vi "OP_Print_TPS_cluster_20170807.vi"() -> ()   [LabVIEW 2013]
uses:
  <userlib>/caLab/Private/Get_PV-1D.vi
  <userlib>/caLab/Private/Get_PV.vi
panel:
  out "x = y?":bool
  out "NOW time":string
  out "NOW date":string
  out "loop2":i32=243
  in  "Save Button":bool
  out "error out 3":errorcluster
  in  "stop":bool
  out "time kickeron":string="kickers"
  out "date kickeron":string="wait to fire"
  out "Cluster":T1={"SR Fill Pattern"=array[864 elements], "Beam Current(mA"=301.91562200000004, "Beam Lifetime(min)"=669.1065769463743, "Beamsize X(um)"=55.54579477590784, "Beamsize Y(um)"=33.648665625479325, "Tune X(from BPM)"=0.1399, "Tune Y(from BPM)"=0.14, "Mode"="Top-Up", "NuX(from BBF) "=0.16718639681347974, "NuY(from BBF)"=0.25219386232318686, "IU22-23gap(R)"=11.0, "IU22-05gap(R)"=7.558, "IU22-05M"=TRUE, "IU22A-09gap(R)"=8.075, "IU22A-09M"=TRUE, "IU22B-09gap(R)"=40.001, "IU22B-09M"=FALSE, "IUT22-21gap(R)"=7.0, "IUT22-21M"=TRUE, "IU22-23M"=TRUE, "IU22A-25gap(R)"=8.18, "IU22A-25M"=TRUE, "IU22B-25gap(R)"=40.0, "IU22B-25M"=FALSE, "EPU48A-41gap(R)"=64.99985000000001, "EPU48A-41gM"=TRUE, "EPU48B-41gap(R)"=65.00399999999999, "EPU48B-41gM"=FALSE, "EPU46-45gap(R)"=45.00005, "EPU46-45gM"=TRUE, "EPU48A-41phase(R)"=0.0001, "EPU48B-41phase(R)"=0.00055, "EPU46-45phase(R)"=0.0, "Grid volt.(V)(S)"=33.0, "Gun mode"="MBM", "Mod.3 HV(kV)(S)"=35.800000000000026, "SR"="SR_DMB_2016_1102_1124LOCO.data", "BR"="Booster_JT_2016_1005_1200.data", "Linac"="Linac2016_1005_0935.data", "LTB"="LTB_JT_2016_1005_1200.data", "BTS"="BTS_2016_1116_1020.data", "RF2 remote"=TRUE, "RF2 OP mode"=TRUE, "RF2 phase.(S)"=-56.70000000000001, "RF Freq.(s)"=499654660.62238467, "RF2 gap volt.(S)"=1400.0, "RF3 remote"=TRUE, "RF3 OP mode"=TRUE, "RF3 phase.(S)"=160.0, "RF3 gap volt.(S)"=1400.0, "BBF V"=TRUE, "BBF H"=TRUE, "BR ext. kicker1(kV)"=18.266, "BR ext. kicker2(kV)"=18.26600000000001, "BR ext. sep.1(V)"=318.8444, "BR ext. sep.2(V)"=444.5, "BR inj. sep.(V)"=105.2, "BR inj. kicker(kV)"=16.40000000000001, "SR kicker4(kV)"=8.27, "SR kicker3(kV)"=8.315, "SR kicker2(kV)"=8.325, "SR kicker1(kV)"=8.4, "SR inj. sep.2(V)"=417.0, "SR inj. sep.1(V)"=419.3416, "Bucket Start"=100.0, "Bucket Last"=630.0, "Bucket Step"=10.0, "Orbit ILK(P)"=TRUE, "IU22-05 Hutch Enable"=TRUE, "IU22A-09M Hutch Enable"=TRUE, "IUT22-21M Hutch Enable"=TRUE, "IU22-23M Hutch Enable"=FALSE, "IU22A-25M Hutch Enable"=TRUE, "EPU48A-41M Hutch Enable"=FALSE, "EPU46-45M Hutch Enable"=TRUE, "EPU46-45 FE Enable"=TRUE, "EPU48A-41 FE Enable"=FALSE, "IU22A-25 FE Enable"=TRUE, "IU22-23 FE Enable"=FALSE, "IUT22-21 FE Enable"=TRUE, "IU22A-09 FE Enable"=TRUE, "IU22-05 FE Enable"=TRUE, "EPU48A-41pM"=TRUE, "EPU48B-41pM"=FALSE, "EPU46-45pM"=FALSE, "Gun volt.(V)(S)"=23.5, "Width count"=30.0, "2ns step"=0.0, "10ps delay"=100.0, "phase shifter"=130.00060000000002, "Taper"=-1.0899999999999999, "05XBPMX 1"=115.877, "09XBPMX 1"=471.421, "21XBPMX 1"=612.331, "23XBPMX 1"=-46.736000000000004, "25XBPMX 1"=462.29900000000004, "41XBPMX 1"=364.139, "45XBPMX 1"=-164.196, "05XBPMY 1"=-62.875, "09XBPMY 1"=-23.034, "21XBPMY 1"=-27.449, "23XBPMY 1"=-89.72200000000001, "25XBPMY 1"=459.291, "41XBPMY 1"=-111.624, "45XBPMY 1"=-57.689, "FOFB H"="On", "FOFB V"="On", "time string"="21:36:25", "date"="2016/11/21", "date (last kicker ON)"="wait to fire", "time string (last kicker ON)"="", "BPMX Graph"={[1, 2, 3, 4, 5, 6, 7, 8, 9, 10, 11, 12, 13, 14, 15, 16, 17, 18, 19, 20, 21, 22, 23, 24, 25, 26, 27, 28, 29, 30, 31, 32, 33, 34, 35, 36, 37, 38, 39, 40, 41, 42, 43, 44, 45, 46, 47, 48, 49, 50, 51, 52, 53, 54, 55, 56, 57, 58, 59, 60, 61, 62, 63, 64, 65, 66, 67, 68, 69, 70, 71, 72, 73, 74, 75, 76, 77, 78, 79, 80, 81, 82, 83, 84, 85, 86, 87, 88, 89, 90, 91, 92, 93, 94, 95, 96, 97, 98, 99, 100, 101, 102, 103, 104, 105, 106, 107, 108, 109, 110, 111, 112, 113, 114, 115, 116, 117, 118, 119, 120, 121, 122, 123, 124, 125, 126, 127, 128, 129, 130, 131, 132, 133, 134, 135, 136, 137, 138, 139, 140, 141, 142, 143, 144, 145, 146, 147, 148, 149, 150, 151, 152, 153, 154, 155, 156, 157, 158, 159, 160, 161, 162, 163, 164, 165, 166, 167, 168, 169, 170, 171, 172, 173, 174], "1rst Value (number)"=[-31.198, -3.303, -73.172, -2.032, 86.386, -75.851, 71.519, -46.03, 6.824, -37.804, 68.275, -4.672, -223.404, -16.867, -6.964, -259.448, -62.697, 1.8880000000000001, 75.267, -92.668, 86.714, -30.843, 12.767, -107.398, -44.436, 161.126, 208.922, 211.488, -27.247, 79.489, 826.962, 470.705, -115.522, -41.497, 159.486, -54.261, -0.64, 42.641, -2.466, -143.394, -24.785, 138.912, -65.805, 42.325, 32.891, -7.298, -96.724, -31.725, 98.531, -80.64, 64.163, 94.83, -44.03, -163.192, 50.589, 46.669000000000004, -87.508, 78.479, 31.618000000000002, -17.077, -125.32600000000001, -3.845, 98.34100000000001, -39.679, 50.247, -58.208, 40.297000000000004, -69.857, 42.548, -19.403, -211.0, -9.082, -322.597, -233.847, -140.75, 97.087, -15.869, -29.053, 59.46, -115.316, 70.896, -60.685, 33.715, 12.09, -520.422, -138.423, -302.753, 79.862, 120.014, 122.671, -55.812, 27.084, 39.115, -138.936, 156.631, 53.777, -72.647, -52.588, 16.002, 45.197, -117.489, 121.709, 27.952, -31.609, -113.58500000000001, 45.019, 55.136, -130.553, 138.93200000000002, 35.998, -30.631, -96.529, -7.589, 100.395, -93.919, 40.569, 79.538, -68.044, -134.578, 2.52, 84.539, -59.166000000000004, 42.576, 34.657000000000004, -15.805, -52.158, 18.484, 4.346, -157.404, 182.672, 202.518, -164.868, -53.871, 8.066, -9.738, -55.594, 92.623, -13.785, 11.587, -60.627, -47.704, 65.516, 57.924, 148.347, -201.348, -302.753, 189.117, 72.681, -134.928, 39.791000000000004, 45.938, -49.072, 54.473, 28.991, -20.657, -80.283, -20.264, 106.907, -121.271, 150.281, -2.243, -11.844, -122.82300000000001, 0.973, 114.186, -107.94, 95.485, 40.314, -36.956, -134.537, 16.196, 91.88, -35.505, -0.018000000000000002]}, "BPMY Graph"={[1, 2, 3, 4, 5, 6, 7, 8, 9, 10, 11, 12, 13, 14, 15, 16, 17, 18, 19, 20, 21, 22, 23, 24, 25, 26, 27, 28, 29, 30, 31, 32, 33, 34, 35, 36, 37, 38, 39, 40, 41, 42, 43, 44, 45, 46, 47, 48, 49, 50, 51, 52, 53, 54, 55, 56, 57, 58, 59, 60, 61, 62, 63, 64, 65, 66, 67, 68, 69, 70, 71, 72, 73, 74, 75, 76, 77, 78, 79, 80, 81, 82, 83, 84, 85, 86, 87, 88, 89, 90, 91, 92, 93, 94, 95, 96, 97, 98, 99, 100, 101, 102, 103, 104, 105, 106, 107, 108, 109, 110, 111, 112, 113, 114, 115, 116, 117, 118, 119, 120, 121, 122, 123, 124, 125, 126, 127, 128, 129, 130, 131, 132, 133, 134, 135, 136, 137, 138, 139, 140, 141, 142, 143, 144, 145, 146, 147, 148, 149, 150, 151, 152, 153, 154, 155, 156, 157, 158, 159, 160, 161, 162, 163, 164, 165, 166, 167, 168, 169, 170, 171, 172, 173, 174], "1rst Value (number)"=[-99.743, 2.851, -30.024, 83.777, -46.733000000000004, -39.889, 2.349, -4.944, 17.022000000000002, 9.824, 11.632, 41.188, -13.992, 13.911, -6.211, 53.857, -48.993, -32.789, -6.3740000000000006, -62.867000000000004, -8.332, 72.09400000000001, -75.398, 53.283, 63.008, -2.23, 43.024, 32.073, -246.641, -93.162, 456.41700000000003, 88.299, 58.803000000000004, 1.7590000000000001, 35.664, 6.575, 18.59, -30.439, 11.254, -28.256, -62.707, -4.503, 1.31, -21.571, 34.77, -8.876, 31.237000000000002, 25.402, 2.726, 20.655, -7.845, -1.443, -31.935000000000002, -16.981, 13.022, 17.515, -82.867, 61.285000000000004, -57.573, 110.363, -27.753, 28.322, -9.241, 53.929, -25.816, 24.231, -57.876, -11.578, 32.087, -70.84, 64.43, 9.409, -157.639, -57.0, 39.267, 30.23, 18.993000000000002, -33.97, 26.195, -10.585, -17.617, -18.667, 31.615000000000002, -25.437, 29.564, 13.537, 6.728, 163.38400000000001, 106.51, -70.056, 12.874, -4.125, -10.855, -21.856, 1.947, 8.096, 11.402000000000001, 5.761, 41.929, -8.752, 18.634, 7.553, -40.034, 39.183, -25.067, -32.557, 5.393, -17.564, -1.614, 20.498, -14.818, 10.313, 35.254, -35.886, 58.359, -36.56, -20.354, 7.593, -21.256, -8.001, -16.79, 10.18, -16.327, 20.416, -10.539, 19.944, -6.801, 13.068, -13.644, 3.468, -0.983, -17.6, 6.785, -26.101, -11.52, 61.191, -32.777, 13.536, 4.026, -14.682, 52.057, -53.883, 27.118000000000002, 31.672, 79.62, 17.715, 15.693, 113.157, -57.095, 14.214, -4.787, -11.148, -3.157, -6.251, -0.764, 3.563, 7.3500000000000005, 10.779, 21.129, 11.36, 7.771, -14.787, -13.278, 0.279, -13.516, -62.422000000000004, -13.389000000000001, 80.56400000000001, -108.465, 69.885, 30.116, 21.421, 32.779, -10.527000000000001]}, "Radio Buttons 2"=enum."absolute", "09XBPMX 2"="", "09XBPMY 2"="", "05XBPMY 2"="", "05XBPMX 2"="", "21XBPMY 2"="", "21XBPMX 2"="", "23XBPMY 2"="", "23XBPMX 2"="", "25XBPMY 2"="", "25XBPMX 2"="", "41XBPMY 2"="", "41XBPMX 2"="", "45XBPMX 2"="", "45XBPMY 2"="", "05 mode"="", "09A mode"="", "09B mode"="", "21 mode"="", "23 mode"="", "25A mode"="", "25B mode"="", "41A mode"="", "41B mode"="", "46 mode"=""} {"45XBPMY 1" format="%#.2f"; "41XBPMY 1" format="%#.2f"; "25XBPMY 1" format="%#.2f"; "23XBPMY 1" format="%#.2f"; "21XBPMY 1" format="%#.2f"; "09XBPMY 1" format="%#.2f"; "05XBPMY 1" format="%#.2f"; "45XBPMX 1" format="%#.2f"; "41XBPMX 1" format="%#.2f"; "25XBPMX 1" format="%#.2f"; "23XBPMX 1" format="%#.2f"; "21XBPMX 1" format="%#.2f"; "09XBPMX 1" format="%#.2f"; "05XBPMX 1" format="%#.2f"; "Taper" format="%#.4f"; "phase shifter" format="%#.3f"; "10ps delay" format="%#.1f"; "2ns step" format="%#.1f"; "Width count" format="%#.1f"; "Gun volt.(V)(S)" format="%#.1f"; "Bucket Step" format="%#.2f"; "Bucket Last" format="%#.2f"; "Bucket Start" format="%#.2f"; "BR ext. kicker1(kV)" format="%#.2f"; "BR ext. kicker2(kV)" format="%#.2f"; "BR ext. sep.1(V)" format="%#.2f"; "BR ext. sep.2(V)" format="%#.2f"; "BR inj. sep.(V)" format="%#.3f"; "BR inj. kicker(kV)" format="%#.3f"; "SR kicker4(kV)" format="%#.2f"; "SR kicker3(kV)" format="%#.2f"; "SR kicker2(kV)" format="%#.2f"; "SR kicker1(kV)" format="%#.2f"; "SR inj. sep.2(V)" format="%#.2f"; "SR inj. sep.1(V)" format="%#.2f"; "RF3 gap volt.(S)" format="%#.0f"; "RF3 phase.(S)" format="%#.1f"; "RF2 gap volt.(S)" format="%#.0f"; "RF Freq.(s)" format="%#.1f"; "RF2 phase.(S)" format="%#.1f"; "Mod.3 HV(kV)(S)" format="%#.3f"; "Grid volt.(V)(S)" format="%#.1f"; "EPU46-45phase(R)" format="%#.4f"; "EPU48B-41phase(R)" format="%#.4f"; "EPU48A-41phase(R)" format="%#.4f"; "EPU46-45gap(R)" format="%#.4f"; "EPU48B-41gap(R)" format="%#.4f"; "EPU48A-41gap(R)" format="%#.4f"; "IU22B-25gap(R)" format="%#.4f"; "IU22A-25gap(R)" format="%#.4f"; "IUT22-21gap(R)" format="%#.4f"; "IU22B-09gap(R)" format="%#.4f"; "IU22A-09gap(R)" format="%#.4f"; "IU22-05gap(R)" format="%#.4f"; "IU22-23gap(R)" format="%#.4f"; "NuY(from BBF)" format="%#.4f"; "NuX(from BBF)" format="%#.4f"; "Tune Y(from BPM)" format="%#.4f"; "Tune X(from BPM)" format="%#.4f"; "Beamsize Y(um)" format="%#.2f"; "Beamsize X(um)" format="%#.2f"; "Beam Lifetime(min)" format="%#.3f"; "Beam Current(mA" format="%#.3f"}
  out "date (last Gun ON)":string="2016/08/29"
  out "time string (last Gun ON)":string="23:28:50"
  out "Value Array (number) 7":dbl[](array[numeric])=[115.877, -62.875, 471.421, -23.034, 612.331, -27.449, -46.736000000000004, -89.72200000000001, 462.29900000000004, 459.291, 364.139, -111.624, -164.196, -57.689]
  out "Value Array (number) 6":dbl[](array[numeric])=[7.558, 8.075, 40.001, 7.0, 11.0, 8.18, 40.0, 64.99985000000001, 0.0001, 65.00399999999999, 0.00055, 45.00005, 0.0, -1.0899999999999999, 130.00060000000002]
  out "1rst Value (string) 2":string[](array[string])=["MBM", "33", "23.5", "350", "35.8", "22485", "22485", "62", "30", "0", "0", "160", "100"]
  out "Value Array (number) 5":dbl[](array[numeric])=[499654641.19275105, 1.0, 0.0, 1335.005102558433, 1400.0, -56.1, 1.0, 0.0, 1362.1066276040413, 1400.0, 160.0]
  out "1rst Value (string)":string[](array[string])=["Linac2016_1005_0935.data", "LTB_JT_2016_1005_1200.data", "Booster_JT_2016_1005_1200.data", "BTS_2016_1116_1020.data", "SR_DMB_2016_1102_1124LOCO.data"]
  out "Value Array (number) 4":dbl[](array[numeric])=[499654660.62238467, 1.0, 0.0, 1334.266859115235, 1400.0, -56.70000000000001, 1.0, 0.0, 1364.570619451613, 1400.0, 160.0]
  out "Value Array (number) 3":dbl[](array[numeric])=[0.0, 33.0, 23.5, 350.0, 35.800000000000026, 22485.0, 22485.0, 62.0, 30.0, 0.0, 0.0, 160.0, 100.0]
  out "Value Array (number) 2":dbl[](array[numeric])=[105.2, 16.40000000000001, 18.266, 18.26600000000001, 318.8444, 444.5, 419.3416, 417.0, 8.4, 8.325, 8.315, 8.27]
  out "Value Array (number)":dbl[](array[numeric])=[1.0, 301.91562200000004, 669.1065769463743, 46.211143740355936, 27.993898190914578, 0.11937377690802348, 0.2162426614481409, 96.68439483642578, 145.84446716308594, 100.0, 630.0, 10.0]
  out "Orbit ILK(A)":bool
  out "Orbit INT. Ang Active":bool
  out "Orbit INT.Ang. On":bool
  out "Orbit INT. Pos Active":bool
  out "Orbit INT.Pos. On":bool
  out "SBM volt.(S)":dbl=350.0 format="%#.1f"
  out "MBM volt.(S)":dbl=23.5 format="%#.1f"
  in  "Copy Button":bool
  in  "Print Button":bool
  in  "Help Button":bool
  in  "Refresh Button":bool
  in  "Open Button":bool
  out "Gun WCM":dbl[](graph)
  out "BR Fill Pattern":dbl[](graph)
  # "TPS OP Handover Information"
  # "Others"
  # "Time："
  # "Valve  Status"
  # "follow"
  # "SM Status"
  # "歷史電流圖\ntrip次數?\n輻射劑量?\n平均氣壓\n目前最高累計劑量\n最近一次觸發時BR電流及WCM數值"
  # "TPS Operational Handover Information v1.2"
  # "SR Status"
  # "Feedback"
  # "Pulse Mag"
  # "LINAC"
  # "x8(ns)"
  # "x2(ns)"
  # "x0.01(ns)"
  # "RF Status"
  # "Hz"
  # "(kV)"
  # "(kV)"
  # "Changeliang@LOP.NSRRC"
  # "SR Fill Pattern"
  # "Lattice Files in using"
  # "ID &Beamline (R)"
  # "mode"
  # "Gap\nmm"
  # "Motor"
  # "Phase"
  # "FE/Hutch"
  # "phase\nshifter"
  # "Taper\n(enc)"
  # "XBPM1X\num"
  # "XBPM1Y\num"
  # "XBPM2X\num"
  # "XBPM2Y\num"
  # "05"
  # "09"
  # "21"
  # "23"
  # "25"
  # "41"
  # "45"
  # "SR Orbit"
  # "BPMX"
  # "BPMY"
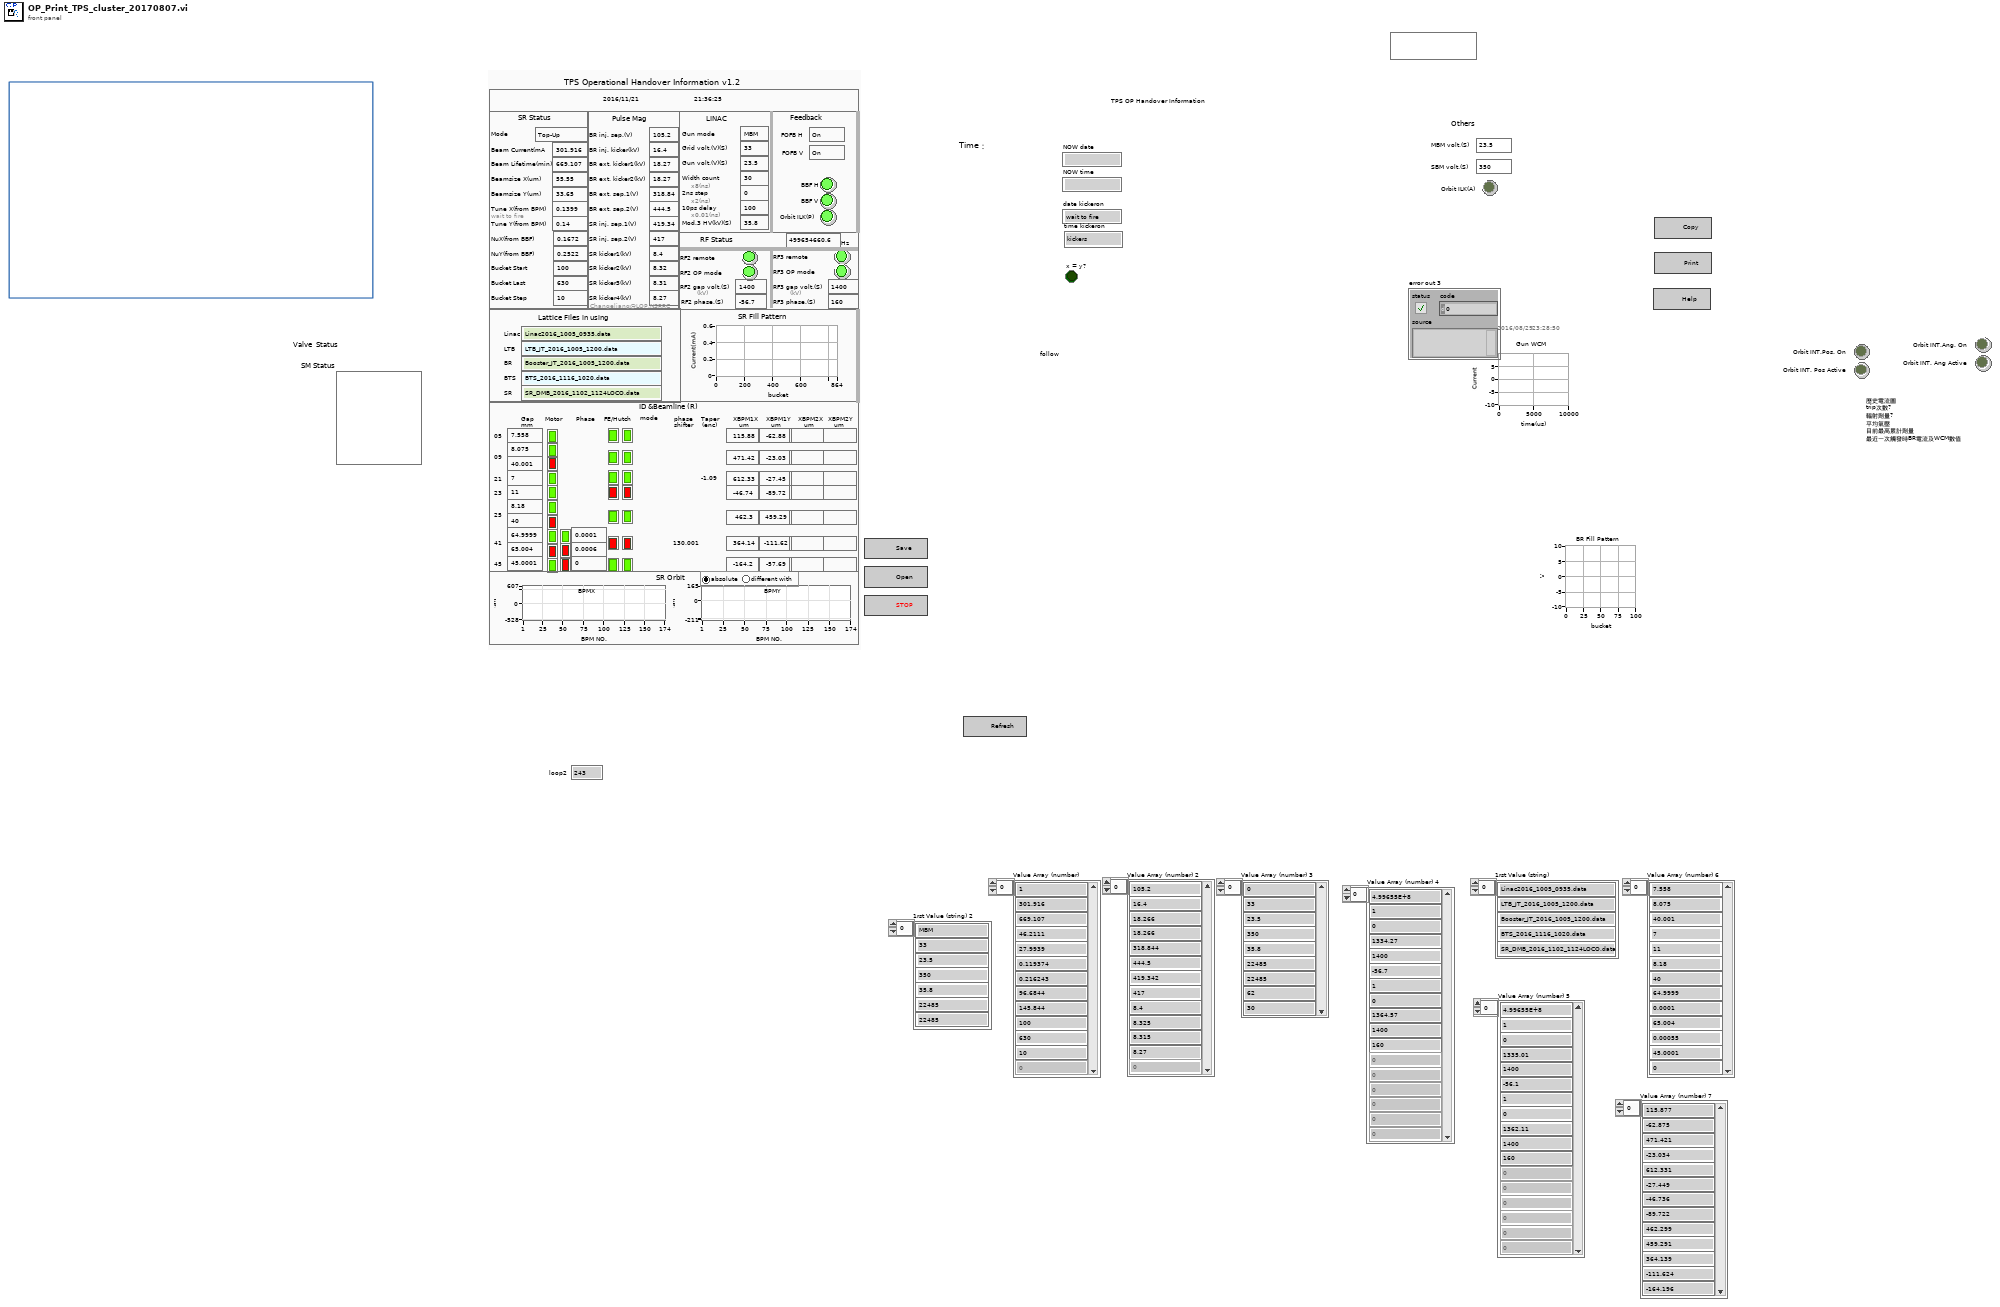
[diagram p1: front panel]
types:
  T1 = cluster{"SR Fill Pattern":dbl[], "Beam Current(mA":dbl, "Beam Lifetime(min)":dbl, "Beamsize X(um)":dbl, "Beamsize Y(um)":dbl, "Tune X(from BPM)":dbl, "Tune Y(from BPM)":dbl, "Mode":string, "NuX(from BBF) ":dbl, "NuY(from BBF)":dbl, "IU22-23gap(R)":dbl, "IU22-05gap(R)":dbl, "IU22-05M":bool, "IU22A-09gap(R)":dbl, "IU22A-09M":bool, "IU22B-09gap(R)":dbl, "IU22B-09M":bool, "IUT22-21gap(R)":dbl, "IUT22-21M":bool, "IU22-23M":bool, "IU22A-25gap(R)":dbl, "IU22A-25M":bool, "IU22B-25gap(R)":dbl, "IU22B-25M":bool, "EPU48A-41gap(R)":dbl, "EPU48A-41gM":bool, "EPU48B-41gap(R)":dbl, "EPU48B-41gM":bool, "EPU46-45gap(R)":dbl, "EPU46-45gM":bool, "EPU48A-41phase(R)":dbl, "EPU48B-41phase(R)":dbl, "EPU46-45phase(R)":dbl, "Grid volt.(V)(S)":dbl, "Gun mode":string, "Mod.3 HV(kV)(S)":dbl, "SR":string, "BR":string, "Linac":string, "LTB":string, "BTS":string, "RF2 remote":bool, "RF2 OP mode":bool, "RF2 phase.(S)":dbl, "RF Freq.(s)":dbl, "RF2 gap volt.(S)":dbl, "RF3 remote":bool, "RF3 OP mode":bool, "RF3 phase.(S)":dbl, "RF3 gap volt.(S)":dbl, "BBF V":bool, "BBF H":bool, "BR ext. kicker1(kV)":dbl, "BR ext. kicker2(kV)":dbl, "BR ext. sep.1(V)":dbl, "BR ext. sep.2(V)":dbl, "BR inj. sep.(V)":dbl, "BR inj. kicker(kV)":dbl, "SR kicker4(kV)":dbl, "SR kicker3(kV)":dbl, "SR kicker2(kV)":dbl, "SR kicker1(kV)":dbl, "SR inj. sep.2(V)":dbl, "SR inj. sep.1(V)":dbl, "Bucket Start":dbl, "Bucket Last":dbl, "Bucket Step":dbl, "Orbit ILK(P)":bool, "IU22-05 Hutch Enable":bool, "IU22A-09M Hutch Enable":bool, "IUT22-21M Hutch Enable":bool, "IU22-23M Hutch Enable":bool, "IU22A-25M Hutch Enable":bool, "EPU48A-41M Hutch Enable":bool, "EPU46-45M Hutch Enable":bool, "EPU46-45 FE Enable":bool, "EPU48A-41 FE Enable":bool, "IU22A-25 FE Enable":bool, "IU22-23 FE Enable":bool, "IUT22-21 FE Enable":bool, "IU22A-09 FE Enable":bool, "IU22-05 FE Enable":bool, "EPU48A-41pM":bool, "EPU48B-41pM":bool, "EPU46-45pM":bool, "Gun volt.(V)(S)":dbl, "Width count":dbl, "2ns step":dbl, "10ps delay":dbl, "phase shifter":dbl, "Taper":dbl, "05XBPMX 1":dbl, "09XBPMX 1":dbl, "21XBPMX 1":dbl, "23XBPMX 1":dbl, "25XBPMX 1":dbl, "41XBPMX 1":dbl, "45XBPMX 1":dbl, "05XBPMY 1":dbl, "09XBPMY 1":dbl, "21XBPMY 1":dbl, "23XBPMY 1":dbl, "25XBPMY 1":dbl, "41XBPMY 1":dbl, "45XBPMY 1":dbl, "FOFB H":string, "FOFB V":string, "time string":string, "date":string, "date (last kicker ON)":string, "time string (last kicker ON)":string, "BPMX Graph":cluster{i32[], "1rst Value (number)":dbl[]}, "BPMY Graph":cluster{i32[], "1rst Value (number)":dbl[]}, "Radio Buttons 2":enum32{"absolute", "different with"}, "09XBPMX 2":string, "09XBPMY 2":string, "05XBPMY 2":string, "05XBPMX 2":string, "21XBPMY 2":string, "21XBPMX 2":string, "23XBPMY 2":string, "23XBPMX 2":string, "25XBPMY 2":string, "25XBPMX 2":string, "41XBPMY 2":string, "41XBPMX 2":string, "45XBPMX 2":string, "45XBPMY 2":string, "05 mode":string, "09A mode":string, "09B mode":string, "21 mode":string, "23 mode":string, "25A mode":string, "25B mode":string, "41A mode":string, "41B mode":string, "46 mode":string}
  T2 = typedef "imagedata.ctl" = cluster{"image type":i32, "image depth":i32, "image":u8[], "mask":u8[], "colors":u32[], "Rectangle":cluster{"left":i16, "top":i16, "right":i16, "bottom":i16}}
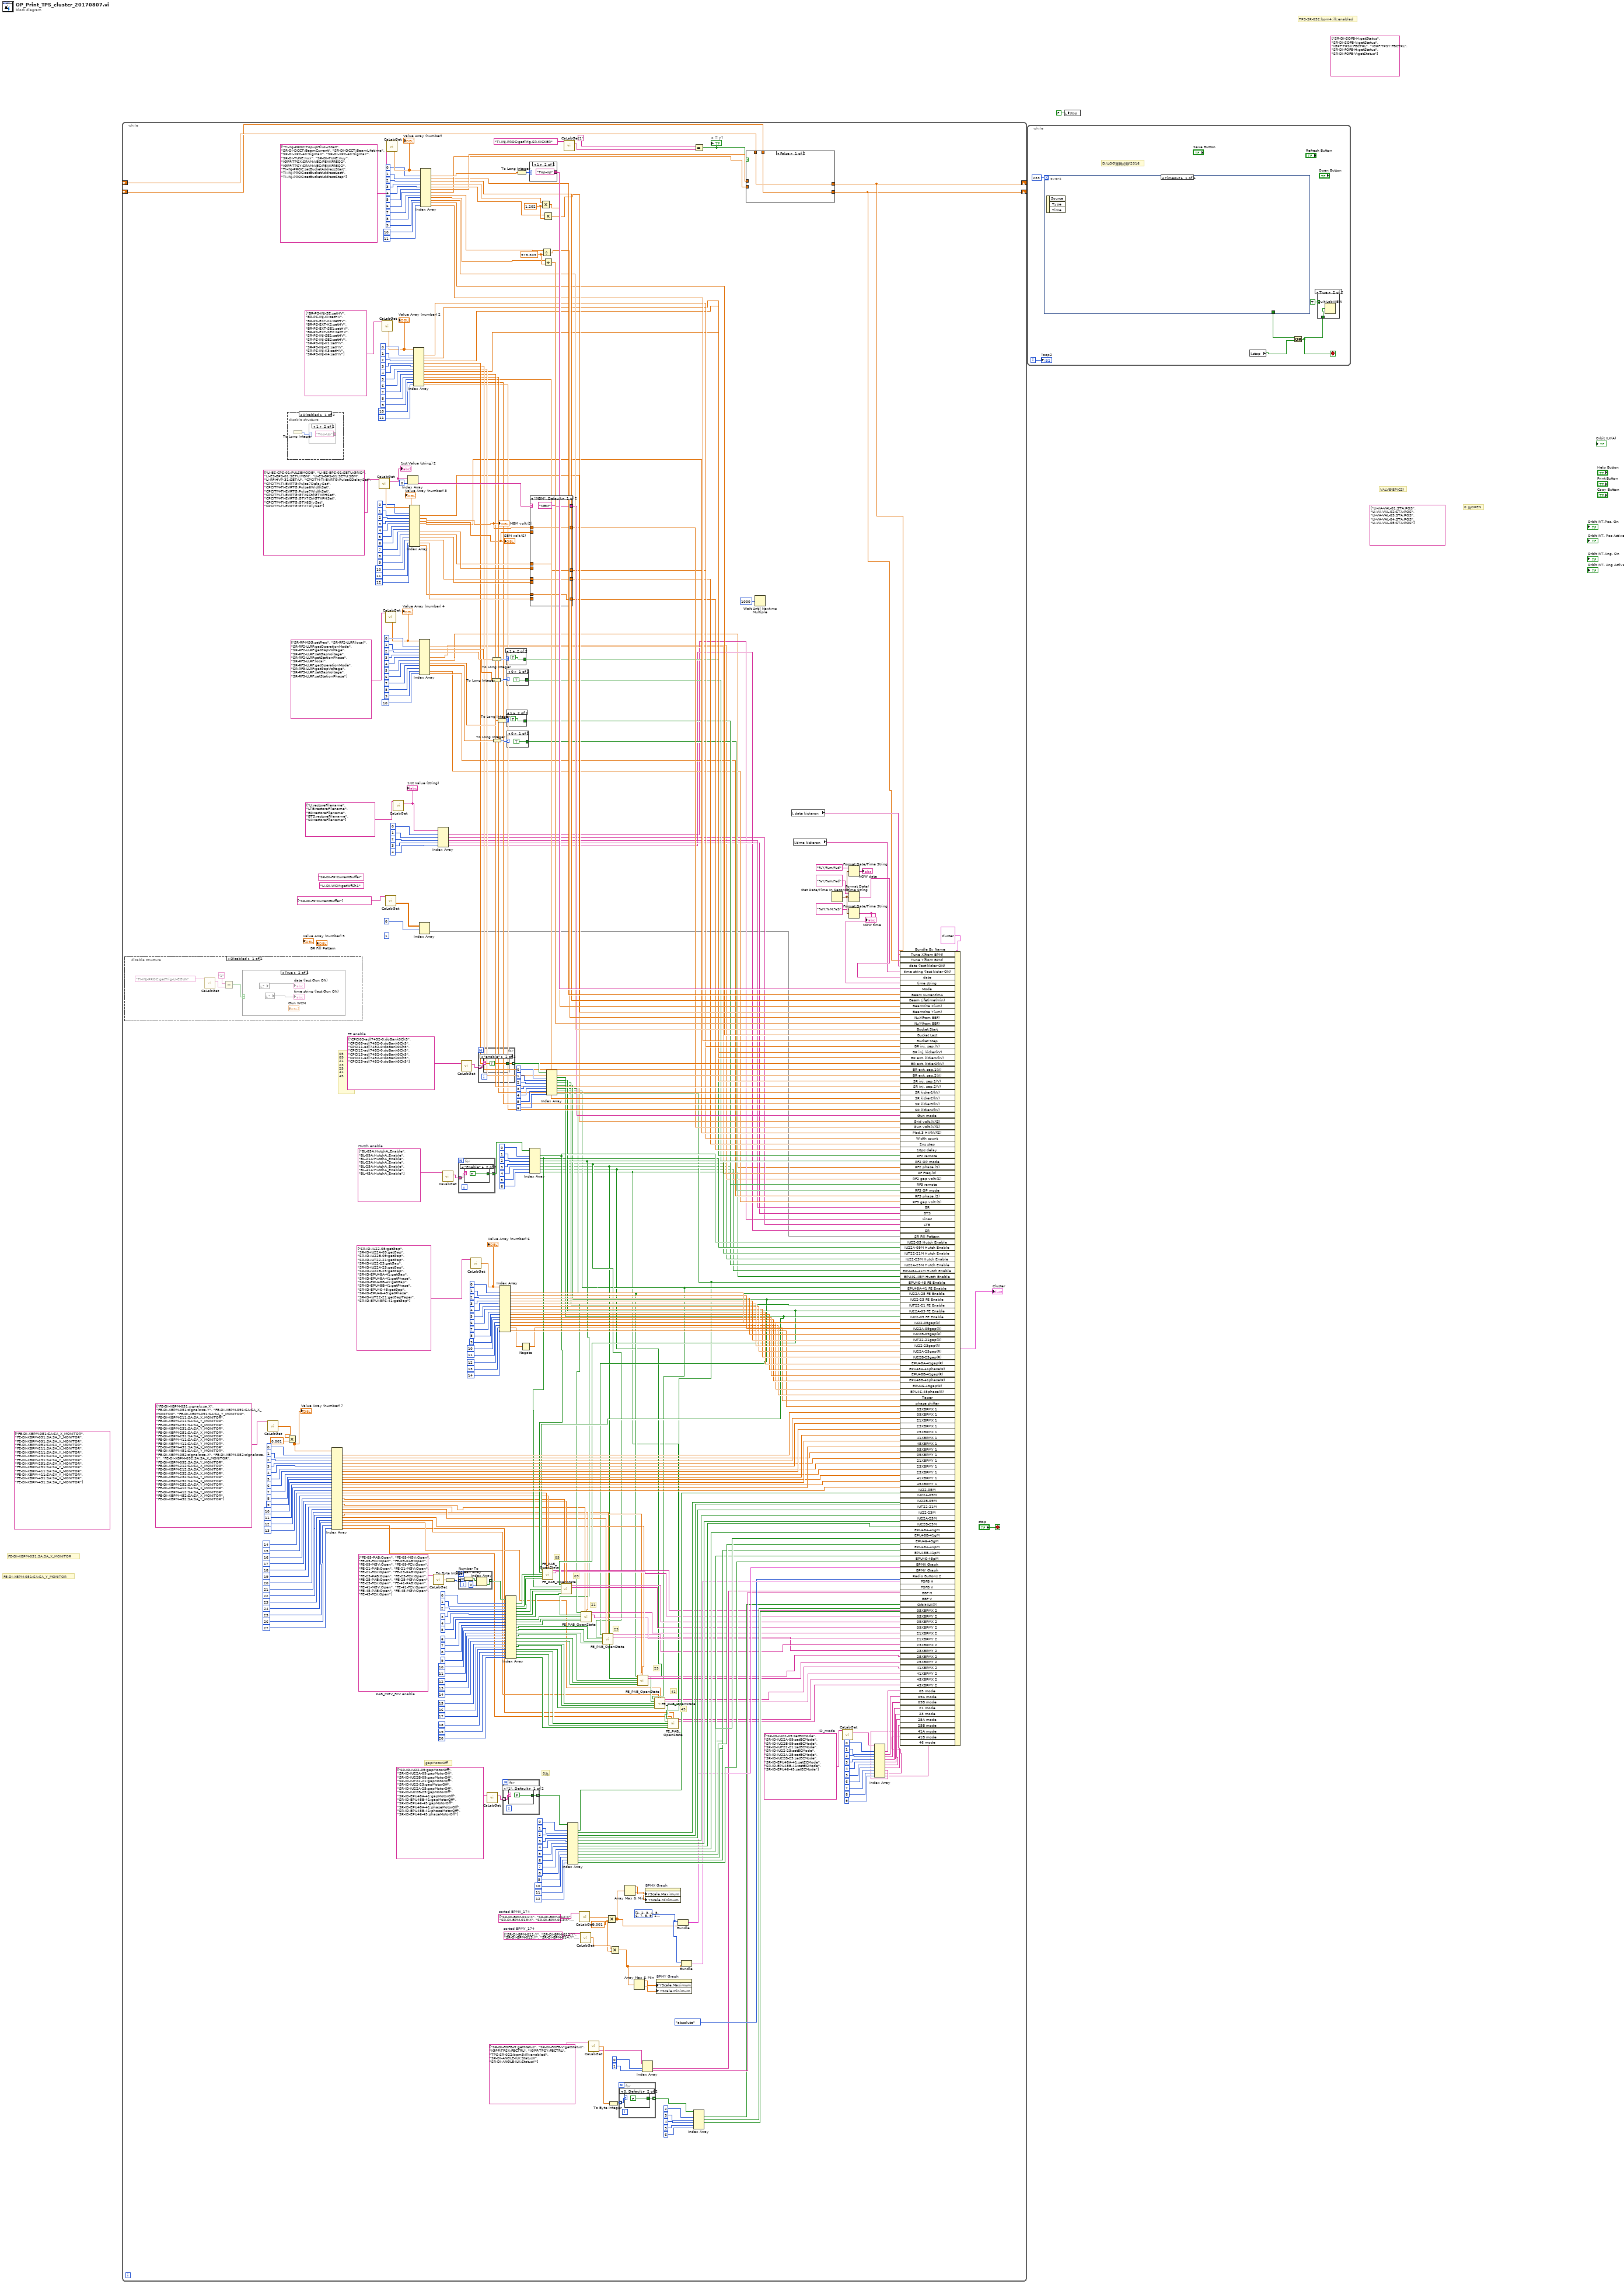
[diagram p0: block diagram]
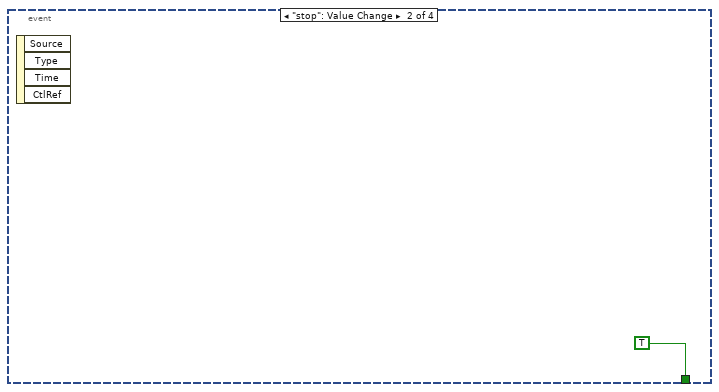
[diagram p3: hidden frame]
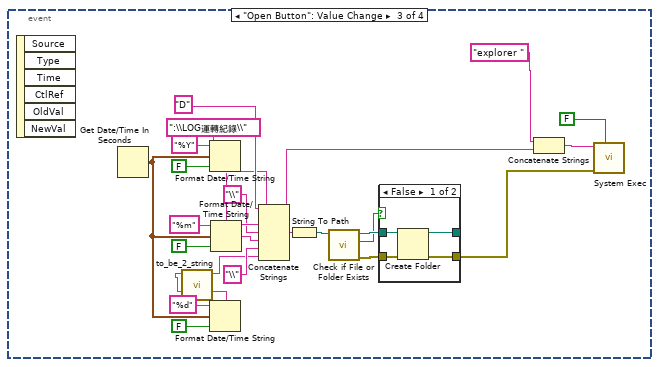
[diagram p4: hidden frame]
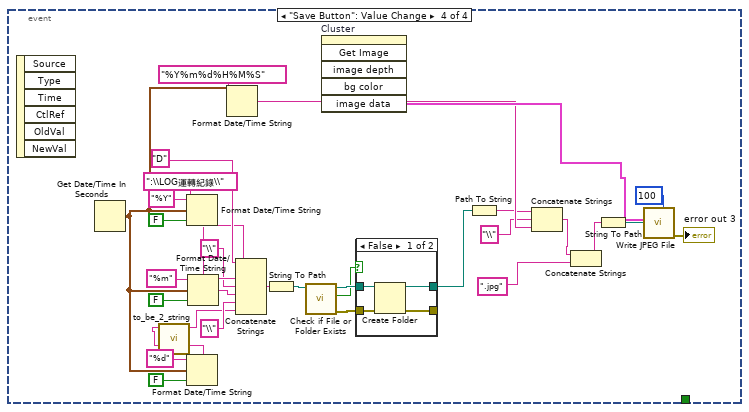
[diagram p6: hidden frame]
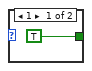
[diagram p8: hidden frame]
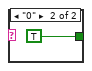
[diagram p11: hidden frame]
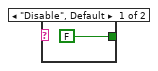
[diagram p12: hidden frame]
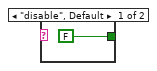
[diagram p13: hidden frame]
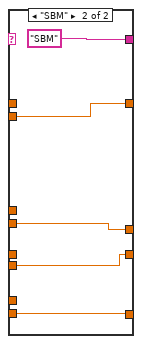
[diagram p14: hidden frame]
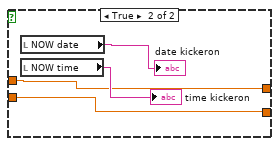
[diagram p15: hidden frame]
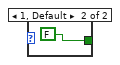
[diagram p16: hidden frame]
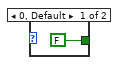
[diagram p17: hidden frame]
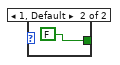
[diagram p18: hidden frame]
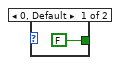
[diagram p19: hidden frame]
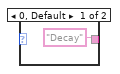
[diagram p20: hidden frame]
diagram:
  (unwired) string[] ["FE-DI-XBPM-051:SA:SA_X_MONITOR", "FE-DI-XBPM-051:SA:SA_Y_MONITOR", "FE-DI-XBPM-091:SA:SA_X_MONITOR", "FE-DI-XBPM-091:SA:SA_Y_MONITOR", "FE-DI-XBPM-211:SA:SA_X_MONITOR", "FE-DI-XBPM-211:SA:SA_Y_MONITOR", "FE-DI-XBPM-231:SA:SA_X_MONITOR", "FE-DI-XBPM-231:SA:SA_Y_MONITOR", "FE-DI-XBPM-251:SA:SA_X_MONITOR", "FE-DI-XBPM-251:SA:SA_Y_MONITOR", "FE-DI-XBPM-411:SA:SA_X_MONITOR", "FE-DI-XBPM-411:SA:SA_Y_MONITOR", "FE-DI-XBPM-451:SA:SA_X_MONITOR", "FE-DI-XBPM-451:SA:SA_Y_MONITOR"]
  (unwired) string[] ["LI-VA-VAL-01:STA:POS", "LI-VA-VAL-02:STA:POS", "LI-VA-VAL-03:STA:POS", "LI-VA-VAL-04:STA:POS", "LI-VA-VAL-05:STA:POS"]
  (unwired) string[] ["SR-DI-SOFB-H:getStatus", "SR-DI-SOFB-V:getStatus", "IGPF:TPSX:FBCTRL", "IGPF:TPSY:FBCTRL", "SR-DI-FOFB-H:getStatus", "SR-DI-FOFB-V:getStatus"]
  # "FE-DI-XBPM-051:SA:SA_Y_MONITOR"
  # "FE-DI-XBPM-051:SA:SA_X_MONITOR"
  # "TPS-SR-052:bpm4:ilk:enabled"
  # "0 為OPEN"
  # "VALVE(EPICS)"
  n1 = while {
    shift-right: [w138] -> _
    shift-left: _ -> [w136]
    shift-right: [w137] -> _
    shift-left: _ -> [w135]
    stop <- "stop" stop-if-true
    w23 = string[] ["SR-ID-IU22-05:setECMode", "SR-ID-IU22A-09:setECMode", "SR-ID-IU22B-09:setECMode", "SR-ID-IUT22-21:setECMode", "SR-ID-IU22-23:setECMode", "SR-ID-IU22A-25:setECMode", "SR-ID-IU22B-25:setECMode", "SR-ID-EPU48A-41:setECMode", "SR-ID-EPU48B-41:setECMode", "SR-ID-EPU46-45:setECMode"]  # ID_mode
    w111 = string[] ["FE-05-PAB:Open", "FE-05-MGV:Open", "FE-05-FCV:Open", "FE-09-PAB:Open", "FE-09-MGV:Open", "FE-09-FCV:Open", "FE-21-PAB:Open", "FE-21-MGV:Open", "FE-21-FCV:Open", "FE-23-PAB:Open", "FE-23-PAB:Open", "FE-23-FCV:Open", "FE-25-PAB:Open", "FE-25-MGV:Open", "FE-25-FCV:Open", "FE-41-PAB:Open", "FE-41-MGV:Open", "FE-41-FCV:Open", "FE-45-PAB:Open", "FE-45-MGV:Open", "FE-45-FCV:Open"]  # PAB_MGV_FCV enable
    (unwired) "LI-DI-WCM:getWfCh1"
    (unwired) "SR-DI-FP:CurrentBuffer"
    w258 = i32[] [1, 2, 3, 4, 5, 6, 7, 8, 9, 10, 11, 12, 13, 14, 15, 16, 17, 18, 19, 20, 21, 22, 23, 24, 25, 26, 27, 28, 29, 30, 31, 32, 33, 34, 35, 36, 37, 38, 39, 40, 41, 42, 43, 44, 45, 46, 47, 48, 49, 50, 51, 52, 53, 54, 55, 56, 57, 58, 59, 60, 61, 62, 63, 64, 65, 66, 67, 68, 69, 70, 71, 72, 73, 74, 75, 76, 77, 78, 79, 80, 81, 82, 83, 84, 85, 86, 87, 88, 89, 90, 91, 92, 93, 94, 95, 96, 97, 98, 99, 100, 101, 102, 103, 104, 105, 106, 107, 108, 109, 110, 111, 112, 113, 114, 115, 116, 117, 118, 119, 120, 121, 122, 123, 124, 125, 126, 127, 128, 129, 130, 131, 132, 133, 134, 135, 136, 137, 138, 139, 140, 141, 142, 143, 144, 145, 146, 147, 148, 149, 150, 151, 152, 153, 154, 155, 156, 157, 158, 159, 160, 161, 162, 163, 164, 165, 166, 167, 168, 169, 170, 171, 172, 173, 174] ("Array 4")
    w256 = 0.001
    w254 = string[] ["SR-DI-BPM-011:Y", "SR-DI-BPM-012:Y", "SR-DI-BPM-013:Y", "SR-DI-BPM-014:Y", "SR-DI-BPM-015:Y", "SR-DI-BPM-016:Y", "SR-DI-BPM-017:Y", "SR-DI-BPM-021:Y", "SR-DI-BPM-022:Y", "SR-DI-BPM-023:Y", "SR-DI-BPM-024:Y", "SR-DI-BPM-025:Y", "SR-DI-BPM-026:Y", "SR-DI-BPM-027:Y", "SR-DI-BPM-031:Y", "SR-DI-BPM-032:Y", "SR-DI-BPM-033:Y", "SR-DI-BPM-034:Y", "SR-DI-BPM-035:Y", "SR-DI-BPM-036:Y", "SR-DI-BPM-037:Y", "SR-DI-BPM-041:Y", "SR-DI-BPM-042:Y", "SR-DI-BPM-043:Y", "SR-DI-BPM-044:Y", "SR-DI-BPM-045:Y", "SR-DI-BPM-046:Y", "SR-DI-BPM-047:Y", "SR-DI-BPM-048:Y", "SR-DI-BPM-050:Y", "SR-DI-BPM-051:Y", "SR-DI-BPM-052:Y", "SR-DI-BPM-053:Y", "SR-DI-BPM-054:Y", "SR-DI-BPM-055:Y", "SR-DI-BPM-056:Y", "SR-DI-BPM-057:Y", "SR-DI-BPM-061:Y", "SR-DI-BPM-062:Y", "SR-DI-BPM-063:Y", "SR-DI-BPM-064:Y", "SR-DI-BPM-065:Y", "SR-DI-BPM-066:Y", "SR-DI-BPM-067:Y", "SR-DI-BPM-071:Y", "SR-DI-BPM-072:Y", "SR-DI-BPM-073:Y", "SR-DI-BPM-074:Y", "SR-DI-BPM-075:Y", "SR-DI-BPM-076:Y", "SR-DI-BPM-077:Y", "SR-DI-BPM-081:Y", "SR-DI-BPM-082:Y", "SR-DI-BPM-083:Y", "SR-DI-BPM-084:Y", "SR-DI-BPM-085:Y", "SR-DI-BPM-086:Y", "SR-DI-BPM-087:Y", "SR-DI-BPM-091:Y", "SR-DI-BPM-092:Y", "SR-DI-BPM-093:Y", "SR-DI-BPM-094:Y", "SR-DI-BPM-095:Y", "SR-DI-BPM-096:Y", "SR-DI-BPM-097:Y", "SR-DI-BPM-101:Y", "SR-DI-BPM-102:Y", "SR-DI-BPM-103:Y", "SR-DI-BPM-104:Y", "SR-DI-BPM-105:Y", "SR-DI-BPM-106:Y", "SR-DI-BPM-107:Y", "SR-DI-BPM-111:Y", "SR-DI-BPM-112:Y", "SR-DI-BPM-113:Y", "SR-DI-BPM-114:Y", "SR-DI-BPM-115:Y", "SR-DI-BPM-116:Y", "SR-DI-BPM-117:Y", "SR-DI-BPM-121:Y", "SR-DI-BPM-122:Y", "SR-DI-BPM-123:Y", "SR-DI-BPM-124:Y", "SR-DI-BPM-125:Y", "SR-DI-BPM-126:Y", "SR-DI-BPM-127:Y", "SR-DI-BPM-128:Y", "SR-DI-BPM-130:Y", "SR-DI-BPM-131:Y", "SR-DI-BPM-132:Y", "SR-DI-BPM-133:Y", "SR-DI-BPM-134:Y", "SR-DI-BPM-135:Y", "SR-DI-BPM-136:Y", "SR-DI-BPM-137:Y", "SR-DI-BPM-141:Y", "SR-DI-BPM-142:Y", "SR-DI-BPM-143:Y", "SR-DI-BPM-144:Y", "SR-DI-BPM-145:Y", "SR-DI-BPM-146:Y", "SR-DI-BPM-147:Y", "SR-DI-BPM-151:Y", "SR-DI-BPM-152:Y", "SR-DI-BPM-153:Y", "SR-DI-BPM-154:Y", "SR-DI-BPM-155:Y", "SR-DI-BPM-156:Y", "SR-DI-BPM-157:Y", "SR-DI-BPM-161:Y", "SR-DI-BPM-162:Y", "SR-DI-BPM-163:Y", "SR-DI-BPM-164:Y", "SR-DI-BPM-165:Y", "SR-DI-BPM-166:Y", "SR-DI-BPM-167:Y", "SR-DI-BPM-171:Y", "SR-DI-BPM-172:Y", "SR-DI-BPM-173:Y", "SR-DI-BPM-174:Y", "SR-DI-BPM-175:Y", "SR-DI-BPM-176:Y", "SR-DI-BPM-177:Y", "SR-DI-BPM-181:Y", "SR-DI-BPM-182:Y", "SR-DI-BPM-183:Y", "SR-DI-BPM-184:Y", "SR-DI-BPM-185:Y", "SR-DI-BPM-186:Y", "SR-DI-BPM-187:Y", "SR-DI-BPM-191:Y", "SR-DI-BPM-192:Y", "SR-DI-BPM-193:Y", "SR-DI-BPM-194:Y", "SR-DI-BPM-195:Y", "SR-DI-BPM-196:Y", "SR-DI-BPM-197:Y", "SR-DI-BPM-201:Y", "SR-DI-BPM-202:Y", "SR-DI-BPM-203:Y", "SR-DI-BPM-204:Y", "SR-DI-BPM-205:Y", "SR-DI-BPM-206:Y", "SR-DI-BPM-207:Y", "SR-DI-BPM-208:Y", "SR-DI-BPM-210:Y", "SR-DI-BPM-211:Y", "SR-DI-BPM-212:Y", "SR-DI-BPM-213:Y", "SR-DI-BPM-214:Y", "SR-DI-BPM-215:Y", "SR-DI-BPM-216:Y", "SR-DI-BPM-217:Y", "SR-DI-BPM-221:Y", "SR-DI-BPM-222:Y", "SR-DI-BPM-223:Y", "SR-DI-BPM-224:Y", "SR-DI-BPM-225:Y", "SR-DI-BPM-226:Y", "SR-DI-BPM-227:Y", "SR-DI-BPM-231:Y", "SR-DI-BPM-232:Y", "SR-DI-BPM-233:Y", "SR-DI-BPM-234:Y", "SR-DI-BPM-235:Y", "SR-DI-BPM-236:Y", "SR-DI-BPM-237:Y", "SR-DI-BPM-241:Y", "SR-DI-BPM-242:Y", "SR-DI-BPM-243:Y", "SR-DI-BPM-244:Y", "SR-DI-BPM-245:Y", "SR-DI-BPM-246:Y", "SR-DI-BPM-247:Y"]  # sorted BPMY_174
    w253 = string[] ["SR-DI-BPM-011:X", "SR-DI-BPM-012:X", "SR-DI-BPM-013:X", "SR-DI-BPM-014:X", "SR-DI-BPM-015:X", "SR-DI-BPM-016:X", "SR-DI-BPM-017:X", "SR-DI-BPM-021:X", "SR-DI-BPM-022:X", "SR-DI-BPM-023:X", "SR-DI-BPM-024:X", "SR-DI-BPM-025:X", "SR-DI-BPM-026:X", "SR-DI-BPM-027:X", "SR-DI-BPM-031:X", "SR-DI-BPM-032:X", "SR-DI-BPM-033:X", "SR-DI-BPM-034:X", "SR-DI-BPM-035:X", "SR-DI-BPM-036:X", "SR-DI-BPM-037:X", "SR-DI-BPM-041:X", "SR-DI-BPM-042:X", "SR-DI-BPM-043:X", "SR-DI-BPM-044:X", "SR-DI-BPM-045:X", "SR-DI-BPM-046:X", "SR-DI-BPM-047:X", "SR-DI-BPM-048:X", "SR-DI-BPM-050:X", "SR-DI-BPM-051:X", "SR-DI-BPM-052:X", "SR-DI-BPM-053:X", "SR-DI-BPM-054:X", "SR-DI-BPM-055:X", "SR-DI-BPM-056:X", "SR-DI-BPM-057:X", "SR-DI-BPM-061:X", "SR-DI-BPM-062:X", "SR-DI-BPM-063:X", "SR-DI-BPM-064:X", "SR-DI-BPM-065:X", "SR-DI-BPM-066:X", "SR-DI-BPM-067:X", "SR-DI-BPM-071:X", "SR-DI-BPM-072:X", "SR-DI-BPM-073:X", "SR-DI-BPM-074:X", "SR-DI-BPM-075:X", "SR-DI-BPM-076:X", "SR-DI-BPM-077:X", "SR-DI-BPM-081:X", "SR-DI-BPM-082:X", "SR-DI-BPM-083:X", "SR-DI-BPM-084:X", "SR-DI-BPM-085:X", "SR-DI-BPM-086:X", "SR-DI-BPM-087:X", "SR-DI-BPM-091:X", "SR-DI-BPM-092:X", "SR-DI-BPM-093:X", "SR-DI-BPM-094:X", "SR-DI-BPM-095:X", "SR-DI-BPM-096:X", "SR-DI-BPM-097:X", "SR-DI-BPM-101:X", "SR-DI-BPM-102:X", "SR-DI-BPM-103:X", "SR-DI-BPM-104:X", "SR-DI-BPM-105:X", "SR-DI-BPM-106:X", "SR-DI-BPM-107:X", "SR-DI-BPM-111:X", "SR-DI-BPM-112:X", "SR-DI-BPM-113:X", "SR-DI-BPM-114:X", "SR-DI-BPM-115:X", "SR-DI-BPM-116:X", "SR-DI-BPM-117:X", "SR-DI-BPM-121:X", "SR-DI-BPM-122:X", "SR-DI-BPM-123:X", "SR-DI-BPM-124:X", "SR-DI-BPM-125:X", "SR-DI-BPM-126:X", "SR-DI-BPM-127:X", "SR-DI-BPM-128:X", "SR-DI-BPM-130:X", "SR-DI-BPM-131:X", "SR-DI-BPM-132:X", "SR-DI-BPM-133:X", "SR-DI-BPM-134:X", "SR-DI-BPM-135:X", "SR-DI-BPM-136:X", "SR-DI-BPM-137:X", "SR-DI-BPM-141:X", "SR-DI-BPM-142:X", "SR-DI-BPM-143:X", "SR-DI-BPM-144:X", "SR-DI-BPM-145:X", "SR-DI-BPM-146:X", "SR-DI-BPM-147:X", "SR-DI-BPM-151:X", "SR-DI-BPM-152:X", "SR-DI-BPM-153:X", "SR-DI-BPM-154:X", "SR-DI-BPM-155:X", "SR-DI-BPM-156:X", "SR-DI-BPM-157:X", "SR-DI-BPM-161:X", "SR-DI-BPM-162:X", "SR-DI-BPM-163:X", "SR-DI-BPM-164:X", "SR-DI-BPM-165:X", "SR-DI-BPM-166:X", "SR-DI-BPM-167:X", "SR-DI-BPM-171:X", "SR-DI-BPM-172:X", "SR-DI-BPM-173:X", "SR-DI-BPM-174:X", "SR-DI-BPM-175:X", "SR-DI-BPM-176:X", "SR-DI-BPM-177:X", "SR-DI-BPM-181:X", "SR-DI-BPM-182:X", "SR-DI-BPM-183:X", "SR-DI-BPM-184:X", "SR-DI-BPM-185:X", "SR-DI-BPM-186:X", "SR-DI-BPM-187:X", "SR-DI-BPM-191:X", "SR-DI-BPM-192:X", "SR-DI-BPM-193:X", "SR-DI-BPM-194:X", "SR-DI-BPM-195:X", "SR-DI-BPM-196:X", "SR-DI-BPM-197:X", "SR-DI-BPM-201:X", "SR-DI-BPM-202:X", "SR-DI-BPM-203:X", "SR-DI-BPM-204:X", "SR-DI-BPM-205:X", "SR-DI-BPM-206:X", "SR-DI-BPM-207:X", "SR-DI-BPM-208:X", "SR-DI-BPM-210:X", "SR-DI-BPM-211:X", "SR-DI-BPM-212:X", "SR-DI-BPM-213:X", "SR-DI-BPM-214:X", "SR-DI-BPM-215:X", "SR-DI-BPM-216:X", "SR-DI-BPM-217:X", "SR-DI-BPM-221:X", "SR-DI-BPM-222:X", "SR-DI-BPM-223:X", "SR-DI-BPM-224:X", "SR-DI-BPM-225:X", "SR-DI-BPM-226:X", "SR-DI-BPM-227:X", "SR-DI-BPM-231:X", "SR-DI-BPM-232:X", "SR-DI-BPM-233:X", "SR-DI-BPM-234:X", "SR-DI-BPM-235:X", "SR-DI-BPM-236:X", "SR-DI-BPM-237:X", "SR-DI-BPM-241:X", "SR-DI-BPM-242:X", "SR-DI-BPM-243:X", "SR-DI-BPM-244:X", "SR-DI-BPM-245:X", "SR-DI-BPM-246:X", "SR-DI-BPM-247:X"]  # sorted BPMX_174
    w313 = string[] ["BL-05A:HutchA_Enable", "BL-09A:HutchA_Enable", "BL-21A:HutchA_Enable", "BL-23A:HutchA_Enable", "BL-25A:HutchA_Enable", "BL-41A:HutchA_Enable", "BL-45A:HutchA_Enable"]  # Hutch enable
    w332 = string[] ["CPCI03-adl7452-0:doBank0Ch5", "CPCI05-adl7452-0:doBank0Ch5", "CPCI11-adl7452-0:doBank0Ch5", "CPCI12-adl7452-0:doBank0Ch5", "CPCI13-adl7452-0:doBank0Ch5", "CPCI21-adl7452-0:doBank0Ch5", "CPCI23-adl7452-0:doBank0Ch5"]  # FE enable
    (unwired) 1 ("index")
    w409 = 578.303 ("y")
    w414 = 1.202 ("y")
    # "45"
    # "41"
    # "25"
    # "23"
    # "21"
    # "09"
    # "05"
    # "0為"
    # "05\n09\n21\n23\n25\n41\n45"
    # "gapMotorOff"
    n2 = disable-structure shown="Disabled" {
      frame Disabled {
        n3 = call-poly <userlib>:"CaLabGet.vi"("PV Name"="TI-INJ-PROC:getTrig-LI-EGUN") -> ("1rst Value (string)"=w442:string)  [unwired: 8 in, 6 out]
        n4 = Equal?(x="1" ("1rst Value (string)"), y=w442) -> (x = y?=w440:bool)
        n5 = case shown="True" w440 {
          frame False {
          }
          frame True {
            n6 = local read item#-1() -> (→"date (last Gun ON)")
            n7 = local read item#-1() -> (→"time string (last Gun ON)")
          }
        }
      }
      frame Enabled {
      }
    }
    n8 = call-poly <userlib>:"CaLabGet.vi"("PV Names"=string[] ["FE-DI-XBPM-051:signals:sa.X", "FE-DI-XBPM-051:signals:sa.Y", "FE-DI-XBPM-091:SA:SA_X_MONITOR", "FE-DI-XBPM-091:SA:SA_Y_MONITOR", "FE-DI-XBPM-211:SA:SA_X_MONITOR", "FE-DI-XBPM-211:SA:SA_Y_MONITOR", "FE-DI-XBPM-231:SA:SA_X_MONITOR", "FE-DI-XBPM-231:SA:SA_Y_MONITOR", "FE-DI-XBPM-251:SA:SA_X_MONITOR", "FE-DI-XBPM-251:SA:SA_Y_MONITOR", "FE-DI-XBPM-411:SA:SA_X_MONITOR", "FE-DI-XBPM-411:SA:SA_Y_MONITOR", "FE-DI-XBPM-451:SA:SA_X_MONITOR", "FE-DI-XBPM-451:SA:SA_Y_MONITOR", "FE-DI-XBPM-052:signals:sa.X", "FE-DI-XBPM-052:signals:sa.Y", "FE-DI-XBPM-092:SA:SA_X_MONITOR", "FE-DI-XBPM-092:SA:SA_Y_MONITOR", "FE-DI-XBPM-212:SA:SA_X_MONITOR", "FE-DI-XBPM-212:SA:SA_Y_MONITOR", "FE-DI-XBPM-232:SA:SA_X_MONITOR", "FE-DI-XBPM-232:SA:SA_Y_MONITOR", "FE-DI-XBPM-252:SA:SA_X_MONITOR", "FE-DI-XBPM-252:SA:SA_Y_MONITOR", "FE-DI-XBPM-412:SA:SA_X_MONITOR", "FE-DI-XBPM-412:SA:SA_Y_MONITOR", "FE-DI-XBPM-452:SA:SA_X_MONITOR", "FE-DI-XBPM-452:SA:SA_Y_MONITOR"] ("appended array")) -> ("1rst Value (number)"=w280:dbl[])  [unwired: 8 in, 6 out]
    n9 = Multiply(x=w280, y=0.001) -> (x*y=w279:dbl[])
    "Value Array (number) 7" <- w279
    n10 = disable-structure shown="Disabled" {
      frame Disabled {
        n11 = To Long Integer() -> (32bit integer=w482:i32)  [unwired: 1 in]
        n12 = case shown="1" w482 {
          tunnel: ["Decay" "Top-Up"] -> _
          frame 0, Default {
          }
          frame 1 {
          }
        }
      }
      frame Enabled {
      }
    }
    n13 = Index Array(array=w279, index #1=0 ("index"), index #2=1 ("index"), index #3=2 ("index"), index #4=3 ("index"), index #5=4 ("index"), index #6=5 ("index"), index #7=6 ("index"), index #8=7 ("index"), index #9=8 ("index"), index #10=9 ("index"), index #11=10 ("index"), index #12=11 ("index"), index #13=12 ("index"), index #14=13 ("index"), index #15=14 ("index"), index #16=15 ("index"), index #17=16 ("index"), index #18=17 ("index"), index #19=18 ("index"), index #20=19 ("index"), index #21=20 ("index"), index #22=21 ("index"), index #23=22 ("index"), index #24=23 ("index"), index #25=24 ("index"), index #26=25 ("index"), index #27=26 ("index"), index #28=27 ("index")) -> (element #1=w195:dbl, element #2=w188:dbl, element #3=w194:dbl, element #4=w187:dbl, element #5=w193:dbl, element #6=w186:dbl, element #7=w192:dbl, element #8=w185:dbl, element #9=w191:dbl, element #10=w184:dbl, element #11=w190:dbl, element #12=w183:dbl, element #13=w189:dbl, element #14=w182:dbl, element #15=w81:dbl, element #16=w80:dbl, element #17=w79:dbl, element #18=w78:dbl, element #19=w69:dbl, element #20=w68:dbl, element #21=w63:dbl, element #22=w62:dbl, element #23=w61:dbl, element #24=w60:dbl, element #25=w29:dbl, element #26=w28:dbl, element #27=w27:dbl, element #28=w26:dbl)
    n14 = call-poly <userlib>:"CaLabGet.vi"("PV Names"=string[] ["LI-ES-CPS-01:PULSEMODE", "LI-ES-BPS-01:SETU:GRID", "LI-ES-BPS-01:SETU:MBM", "LI-ES-BPS-01:SETU:SBM", "LI-RF-HVP-31:SET:U", "CPCITM-TI-EVRTG:Pulse6DelaySet", "CPCITM-TI-EVRTG:Pulse7DelaySet", "CPCITM-TI-EVRTG:Pulse6WidthSet", "CPCITM-TI-EVRTG:Pulse7WidthSet", "CPCITM-TI-EVRTG:GTX6CtrlGTXPHSet", "CPCITM-TI-EVRTG:GTX7CtrlGTXPHSet", "CPCITM-TI-EVRTG:GTX6DlySet", "CPCITM-TI-EVRTG:GTX7DlySet"]) -> ("1rst Value (string)"=w342:string[], "1rst Value (number)"=w393:dbl[])  [unwired: 8 in, 5 out]
    "Value Array (number) 3" <- w393
    "1rst Value (string) 2" <- w342
    n15 = call-poly <userlib>:"CaLabGet.vi"("PV Names"=string[] ["BR-PS-INJ-SE:setHV", "BR-PS-INJ-KI:setHV", "BR-PS-EXT-K1:setHV", "BR-PS-EXT-K2:setHV", "BR-PS-EXT-SE1:setHV", "BR-PS-EXT-SE2:setHV", "SR-PS-INJ-SE1:setHV", "SR-PS-INJ-SE2:setHV", "SR-PS-INJ-K1:setHV", "SR-PS-INJ-K2:setHV", "SR-PS-INJ-K3:setHV", "SR-PS-INJ-K4:setHV"]) -> ("1rst Value (number)"=w395:dbl[])  [unwired: 8 in, 6 out]
    "Value Array (number) 2" <- w395
    n16 = call-poly <userlib>:"CaLabGet.vi"("PV Names"=string[] ["SR-RF-MSG:setFreq", "SR-RF2-LLRF:local", "SR-RF2-LLRF:getOperationMode", "SR-RF2-LLRF:getGapVoltage", "SR-RF2-LLRF:setGapVoltage", "SR-RF2-LLRF:setStationPhase", "SR-RF3-LLRF:local", "SR-RF3-LLRF:getOperationMode", "SR-RF3-LLRF:getGapVoltage", "SR-RF3-LLRF:setGapVoltage", "SR-RF3-LLRF:setStationPhase"]) -> ("1rst Value (number)"=w368:dbl[])  [unwired: 8 in, 6 out]
    "Value Array (number) 4" <- w368
    n17 = call-poly <userlib>:"CaLabGet.vi"("PV Names"=string[] ["SR-DI-FP:CurrentBuffer"]) -> ("Value Array (number)"=w350:dbl[][])  [unwired: 8 in, 6 out]
    n18 = call-poly <userlib>:"CaLabGet.vi"("PV Names"=string[] ["TI-INJ-PROC:TopupHiLowStart", "SR-DI-DCCT:BeamCurrent", "SR-DI-DCCT:BeamLifetime", "SR-DI-XPC-40:SigmaX", "SR-DI-XPC-40:SigmaY", "SR-DI-TUNE:nux", "SR-DI-TUNE:nuy", "IGPF:TPSX:SRAM:VEC:PEAKFREQ2", "IGPF:TPSY:SRAM:VEC:PEAKFREQ2", "TI-INJ-PROC:setBucketAddressStart", "TI-INJ-PROC:setBucketAddressLast", "TI-INJ-PROC:setBucketAddressStep"]) -> ("1rst Value (number)"=w429:dbl[])  [unwired: 8 in, 6 out]
    "Value Array (number)" <- w429
    n19 = call-poly <userlib>:"CaLabGet.vi"("PV Names"=string[] ["LI:restoreFilename", "LTB:restoreFilename", "BR:restoreFilename", "BTS:restoreFilename", "SR:restoreFilename"]) -> ("1rst Value (string)"=w352:string[])  [unwired: 8 in, 6 out]
    "1rst Value (string)" <- w352
    n20 = Index Array(array=w342, index=0) -> (element=w340:string)
    n21 = Index Array(array=w393, index #1=0 ("index"), index #2=1 ("index"), index #3=2 ("index"), index #4=3 ("index"), index #5=4 ("index"), index #6=5 ("index"), index #7=6 ("index"), index #8=7 ("index"), index #9=8 ("index"), index #10=9 ("index"), index #11=10 ("index"), index #12=11 ("index"), index #13=12 ("index")) -> (element #2=w228:dbl, element #3=w344:dbl, element #4=w343:dbl, element #5=w226:dbl, element #8=w339:dbl, element #9=w338:dbl, element #10=w337:dbl, element #11=w336:dbl, element #12=w335:dbl, element #13=w334:dbl)  [unwired: 3 out]
    "MBM volt.(S)" <- w344
    "SBM volt.(S)" <- w343
    n22 = Index Array(array=w395, index #1=0 ("index"), index #2=1 ("index"), index #3=2 ("index"), index #4=3 ("index"), index #5=4 ("index"), index #6=5 ("index"), index #7=6 ("index"), index #8=7 ("index"), index #9=8 ("index"), index #10=9 ("index"), index #11=10 ("index"), index #12=11 ("index")) -> (element #1=w241:dbl, element #2=w240:dbl, element #3=w239:dbl, element #4=w238:dbl, element #5=w237:dbl, element #6=w236:dbl, element #7=w235:dbl, element #8=w234:dbl, element #9=w233:dbl, element #10=w232:dbl, element #11=w231:dbl, element #12=w230:dbl)
    n23 = Index Array(array=w368, index #1=0 ("index"), index #2=1 ("index"), index #3=2 ("index"), index #4=3 ("index"), index #5=4 ("index"), index #6=5 ("index"), index #7=6 ("index"), index #8=7 ("index"), index #9=8 ("index"), index #10=9 ("index"), index #11=10 ("index")) -> (element #1=w220:dbl, element #2=w365:dbl, element #3=w363:dbl, element #5=w141:dbl, element #6=w142:dbl, element #7=w360:dbl, element #8=w359:dbl, element #10=w216:dbl, element #11=w217:dbl)  [unwired: 2 out]
    n24 = Index Array(array=w350, index (row)=0 ("index")) -> (element=w210:dbl[])  [unwired: 1 in]
    n25 = Index Array(array=w429, index #1=0 ("index"), index #2=1 ("index"), index #3=2 ("index"), index #4=3 ("index"), index #5=4 ("index"), index #6=5 ("index"), index #7=6 ("index"), index #8=7 ("index"), index #9=8 ("index"), index #10=9 ("index"), index #11=10 ("index"), index #12=11 ("index")) -> (element #1=w427:dbl, element #2=w250:dbl, element #3=w249:dbl, element #4=w415:dbl, element #5=w413:dbl, element #6=w412:dbl, element #7=w411:dbl, element #8=w410:dbl, element #9=w408:dbl, element #10=w244:dbl, element #11=w243:dbl, element #12=w242:dbl)
    n26 = call-poly <userlib>:"CaLabGet.vi"("PV Names"=w111) -> ("1rst Value (number)"=w113:dbl[])  [unwired: 8 in, 6 out]
    n27 = Index Array(array=w352, index #1=0 ("index"), index #2=1 ("index"), index #3=2 ("index"), index #4=3 ("index"), index #5=4 ("index")) -> (element #1=w212:string, element #2=w211:string, element #3=w215:string, element #4=w214:string, element #5=w213:string)
    n28 = call-poly <userlib>:"CaLabGet.vi"("PV Names"=w313) -> ("1rst Value (string)"=w321:string[])  [unwired: 8 in, 6 out]
    n29 = To Byte Integer(number=w113) -> (8bit integer=w112:i8[])
    n30 = for {
      tunnel: w112 -> [w435] mode=indexing
      tunnel: [w432] -> w89 mode=indexing
      n31 = Number To Boolean Array(number=w435) -> (Boolean array=w434:bool[])
      n32 = Index Array(array=w434, index=0) -> (element=w432:bool)
    }
    n33 = for {
      tunnel: w321 -> [w451] mode=indexing
      tunnel: [w450] -> w322 mode=indexing
      n34 = case shown="\"Enable\"" w451 {
        tunnel: [FALSE TRUE] -> w450
        frame "Disable", Default {
        }
        frame "Enable" {
        }
      }
    }
    n35 = call-poly <userlib>:"CaLabGet.vi"("PV Names"=w332) -> ("1rst Value (string)"=w324:string[])  [unwired: 8 in, 6 out]
    n36 = call-poly <userlib>:"CaLabGet.vi"("PV Names"=string[] ["SR-ID-IU22-05:getGap", "SR-ID-IU22A-09:getGap", "SR-ID-IU22B-09:getGap", "SR-ID-IUT22-21:getGap", "SR-ID-IU22-23:getGap", "SR-ID-IU22A-25:getGap", "SR-ID-IU22B-25:getGap", "SR-ID-EPU48A-41:getGap", "SR-ID-EPU48A-41:getPhase", "SR-ID-EPU48B-41:getGap", "SR-ID-EPU48B-41:getPhase", "SR-ID-EPU46-45:getGap", "SR-ID-EPU46-45:getPhase", "SR-ID-IUT22-21:getGapTaper", "SR-ID-EPU48PS-41:getGap"]) -> ("1rst Value (number)"=w312:dbl[])  [unwired: 8 in, 6 out]
    "Value Array (number) 6" <- w312
    n37 = for {
      tunnel: w324 -> [w455] mode=indexing
      tunnel: [w454] -> w323 mode=indexing
      n38 = case shown="\"enable\"" w455 {
        tunnel: [FALSE TRUE] -> w454
        frame "disable", Default {
        }
        frame "enable" {
        }
      }
    }
    n39 = call-poly <userlib>:"CaLabGet.vi"("PV Names"=string[] ["SR-ID-IU22-05:gapMotorOff", "SR-ID-IU22A-09:gapMotorOff", "SR-ID-IU22B-09:gapMotorOff", "SR-ID-IUT22-21:gapMotorOff", "SR-ID-IU22-23:gapMotorOff", "SR-ID-IU22A-25:gapMotorOff", "SR-ID-IU22B-25:gapMotorOff", "SR-ID-EPU48A-41:gapMotorOff", "SR-ID-EPU48B-41:gapMotorOff", "SR-ID-EPU46-45:gapMotorOff", "SR-ID-EPU48A-41:phaseMotorOff", "SR-ID-EPU48B-41:phaseMotorOff", "SR-ID-EPU46-45:phaseMotorOff"]) -> ("1rst Value (string)"=w264:string[])  [unwired: 8 in, 6 out]
    n40 = To Long Integer(number=w363) -> (32bit integer=w364:i32)
    n41 = To Long Integer(number=w365) -> (32bit integer=w366:i32)
    n42 = To Long Integer(number=w359) -> (32bit integer=w362:i32)
    n43 = To Long Integer(number=w360) -> (32bit integer=w361:i32)
    n44 = Index Array(array=w312, index #1=0 ("index"), index #2=1 ("index"), index #3=2 ("index"), index #4=3 ("index"), index #5=4 ("index"), index #6=5 ("index"), index #7=6 ("index"), index #8=7 ("index"), index #9=8 ("index"), index #10=9 ("index"), index #11=10 ("index"), index #12=11 ("index"), index #13=12 ("index"), index #14=13 ("index"), index #15=14 ("index")) -> (element #1=w209:dbl, element #2=w208:dbl, element #3=w207:dbl, element #4=w206:dbl, element #5=w205:dbl, element #6=w204:dbl, element #7=w203:dbl, element #8=w202:dbl, element #9=w201:dbl, element #10=w200:dbl, element #11=w199:dbl, element #12=w198:dbl, element #13=w197:dbl, element #14=w140:dbl, element #15=w196:dbl)
    n45 = for {
      tunnel: w264 -> [w447] mode=indexing
      tunnel: [w446] -> w263 mode=indexing
      n46 = case shown="\"1\", Default" w447 {
        tunnel: [FALSE TRUE] -> w446
        frame "1", Default {
        }
        frame "0" {
        }
      }
    }
    n47 = Index Array(array=w89, index #1=0 ("index"), index #2=1 ("index"), index #3=2 ("index"), index #4=3 ("index"), index #5=4 ("index"), index #6=5 ("index"), index #7=6 ("index"), index #8=7 ("index"), index #9=8 ("index"), index #10=9 ("index"), index #11=10 ("index"), index #12=11 ("index"), index #13=12 ("index"), index #14=13 ("index"), index #15=14 ("index"), index #16=15 ("index"), index #17=16 ("index"), index #18=17 ("index"), index #19=18 ("index"), index #20=19 ("index"), index #21=20 ("index")) -> (element #1=w86:bool, element #2=w85:bool, element #3=w84:bool, element #4=w73:bool, element #5=w72:bool, element #6=w71:bool, element #7=w66:bool, element #8=w65:bool, element #9=w64:bool, element #10=w55:bool, element #11=w54:bool, element #12=w53:bool, element #13=w48:bool, element #14=w47:bool, element #15=w46:bool, element #16=w45:bool, element #17=w44:bool, element #18=w43:bool, element #19=w42:bool, element #20=w41:bool, element #21=w40:bool)
    n48 = case shown="1" w366 {
      tunnel: [FALSE TRUE] -> w222
      frame 0, Default {
      }
      frame 1 {
      }
    }
    n49 = case shown="1" w361 {
      tunnel: [FALSE TRUE] -> w219
      frame 0, Default {
      }
      frame 1 {
      }
    }
    n50 = case shown="0" w364 {
      tunnel: [TRUE FALSE] -> w221
      frame 0 {
      }
      frame 1, Default {
      }
    }
    n51 = case shown="0" w362 {
      tunnel: [TRUE FALSE] -> w218
      frame 0 {
      }
      frame 1, Default {
      }
    }
    n52 = To Long Integer(number=w427) -> (32bit integer=w430:i32)
    n53 = Negate(x=w140) -> (-x=w139:dbl)
    n54 = case shown="1" w430 {
      tunnel: ["Decay" "Top-Up"] -> w251
      frame 0, Default {
      }
      frame 1 {
      }
    }
    n55 = Index Array(array=w322, index #1=0 ("index"), index #2=1 ("index"), index #3=2 ("index"), index #4=3 ("index"), index #5=4 ("index"), index #6=5 ("index"), index #7=6 ("index")) -> (element #1=w87:bool, element #2=w83:bool, element #3=w67:bool, element #4=w50:bool, element #5=w49:bool, element #6=w31:bool, element #7=w30:bool)
    n56 = case shown="\"MBM\", Default" w340 {
      tunnel: ["MBM" "SBM"] -> w229
      tunnel: w344 -> [w461 _]
      tunnel: [w461 w466] -> w227
      tunnel: w343 -> [_ w466]
      tunnel: w339 -> [_ w465]
      tunnel: w338 -> [w460 _]
      tunnel: [w460 w465] -> w225
      tunnel: w337 -> [_ w464]
      tunnel: w336 -> [w459 _]
      tunnel: [w459 w464] -> w224
      tunnel: w335 -> [_ w463]
      tunnel: w334 -> [w458 _]
      tunnel: [w458 w463] -> w223
      frame "MBM", Default {
      }
      frame "SBM" {
      }
    }
    n57 = Multiply(x=w415, y=w414) -> (x*y=w248:dbl)
    n58 = Divide(x=w410, y=w409) -> (x/y=w246:dbl)
    n59 = Multiply(x=w413, y=w414) -> (x*y=w247:dbl)
    n60 = Divide(x=w408, y=w409) -> (x/y=w245:dbl)
    n61 = Index Array(array=w323, index #1=0 ("index"), index #2=1 ("index"), index #3=2 ("index"), index #4=3 ("index"), index #5=4 ("index"), index #6=5 ("index"), index #7=6 ("index")) -> (element #1=w88:bool, element #2=w82:bool, element #3=w70:bool, element #4=w52:bool, element #5=w51:bool, element #6=w33:bool, element #7=w32:bool)
    n62 = call "FE_PAB_OpenState.vi"("FE"=w88, "XBPMX 2"=w81, "XBPMY 2"=w80, "Hutch"=w87, "PAB"=w86, "MGV"=w85, "FCV"=w84) -> ("XBPMX 2"=w77:string, "XBPMY 2"=w76:string)  [unwired: 7 in]
    n63 = call "FE_PAB_OpenState.vi"("FE"=w82, "XBPMX 2"=w79, "XBPMY 2"=w78, "Hutch"=w83, "PAB"=w73, "MGV"=w72, "FCV"=w71) -> ("XBPMX 2"=w75:string, "XBPMY 2"=w74:string)  [unwired: 7 in]
    n64 = call-poly <userlib>:"CaLabGet.vi"("PV Name"="TI-INJ-PROC:getTrig-SR-KICKER") -> ("1rst Value (string)"=w347:string)  [unwired: 8 in, 6 out]
    n65 = Index Array(array=w263, index #1=0 ("index"), index #2=1 ("index"), index #3=2 ("index"), index #4=3 ("index"), index #5=4 ("index"), index #6=5 ("index"), index #7=6 ("index"), index #8=7 ("index"), index #9=8 ("index"), index #10=9 ("index"), index #11=10 ("index"), index #12=11 ("index"), index #13=12 ("index")) -> (element #1=w181:bool, element #2=w180:bool, element #3=w179:bool, element #4=w178:bool, element #5=w177:bool, element #6=w176:bool, element #7=w175:bool, element #8=w174:bool, element #9=w173:bool, element #10=w172:bool, element #11=w171:bool, element #12=w170:bool, element #13=w169:bool)
    n66 = call-poly <userlib>:"CaLabGet.vi"("PV Names"=w253) -> ("1rst Value (number)"=w255:dbl[])  [unwired: 8 in, 6 out]
    n67 = call-poly <userlib>:"CaLabGet.vi"("PV Names"=w254) -> ("1rst Value (number)"=w257:dbl[])  [unwired: 8 in, 6 out]
    n68 = call "FE_PAB_OpenState.vi"("FE"=w70, "XBPMX 2"=w69, "XBPMY 2"=w68, "Hutch"=w67, "PAB"=w66, "MGV"=w65, "FCV"=w64) -> ("XBPMX 2"=w59:string, "XBPMY 2"=w58:string)  [unwired: 7 in]
    n69 = call-poly <userlib>:"CaLabGet.vi"("PV Names"=string[] ["SR-DI-FOFB-H:getStatus", "SR-DI-FOFB-V:getStatus", "IGPF:TPSX:FBCTRL", "IGPF:TPSY:FBCTRL", "TPS-SR-022:bpm3:ilk:enabled", "SR-DI-ANGLE-ILK:StatusX", "SR-DI-ANGLE-ILK:StatusY"]) -> ("1rst Value (string)"=w155:string[], "1rst Value (number)"=w156:dbl[])  [unwired: 8 in, 5 out]
    n70 = call "FE_PAB_OpenState.vi"("FE"=w52, "XBPMX 2"=w63, "XBPMY 2"=w62, "Hutch"=w50, "PAB"=w55, "MGV"=w54, "FCV"=w53) -> ("XBPMX 2"=w57:string, "XBPMY 2"=w56:string)  [unwired: 7 in]
    n71 = Multiply(x=w255, y=w256) -> (x*y=w129:dbl[])
    n72 = To Byte Integer(number=w156) -> (8bit integer=w152:i8[])
    n73 = Multiply(x=w257, y=w256) -> (x*y=w132:dbl[])
    n74 = for {
      tunnel: w152 -> [w437] mode=indexing
      tunnel: [w436] -> w162 mode=indexing
      n75 = case shown="0, Default" w437 {
        tunnel: [TRUE FALSE] -> w436
        frame 1 {
        }
        frame 0, Default {
        }
      }
    }
    n76 = Array Max & Min(array=w129) -> (max value=w131:dbl, min value=w130:dbl)  [unwired: 2 out]
    n77 = Array Max & Min(array=w132) -> (max value=w134:dbl, min value=w133:dbl)  [unwired: 2 out]
    n78 = call "FE_PAB_OpenState.vi"("FE"=w51, "XBPMX 2"=w61, "XBPMY 2"=w60, "Hutch"=w49, "PAB"=w48, "MGV"=w47, "FCV"=w46) -> ("XBPMX 2"=w39:string, "XBPMY 2"=w38:string)  [unwired: 7 in]
    n79 = Index Array(array=w155, index #1=0 ("index"), index #2=1 ("index")) -> (element #1=w150:string, element #2=w149:string)
    n80 = property on="BPMX Graph" class="XYGraph (strict)"("YScale.Maximum"=w131, "YScale.Minimum"=w130) -> ()  [unwired: 2 in, 2 out]
    n81 = call "FE_PAB_OpenState.vi"("FE"=w33, "XBPMX 2"=w29, "XBPMY 2"=w28, "Hutch"=w31, "PAB"=w45, "MGV"=w44, "FCV"=w43) -> ("XBPMX 2"=w37:string, "XBPMY 2"=w36:string)  [unwired: 7 in]
    n82 = property on="BPMY Graph" class="XYGraph (strict)"("YScale.Maximum"=w134, "YScale.Minimum"=w133) -> ()  [unwired: 2 in, 2 out]
    n83 = call "FE_PAB_OpenState.vi"("FE"=w32, "XBPMX 2"=w27, "XBPMY 2"=w26, "Hutch"=w30, "PAB"=w42, "MGV"=w41, "FCV"=w40) -> ("XBPMX 2"=w35:string, "XBPMY 2"=w34:string)  [unwired: 7 in]
    n84 = Bundle("Array 4"=w258, w129) -> (w168:cluster{"Array 4":i32[], dbl[]})  [unwired: 1 in]
    n85 = Bundle("Array 4"=w258, w132) -> (w167:cluster{"Array 4":i32[], dbl[]})  [unwired: 1 in]
    n86 = Index Array(array=w162, index #1=2 ("index"), index #2=3 ("index"), index #3=4 ("index"), index #4=5 ("index"), index #5=6 ("index")) -> (element #1=w148:bool, element #2=w147:bool, element #3=w146:bool)  [unwired: 2 out]
    n87 = Equal?(x="1" ("1rst Value (string)"), y=w347) -> (x = y?=w345:bool)
    "x = y?" <- w345
    n88 = case shown="False" w345 {
      tunnel: w412 -> [_ w471]
      tunnel: w411 -> [_ w470]
      tunnel: [w469 w471] -> w138
      tunnel: [w468 w470] -> w137
      tunnel: w136 -> [w469 _]
      tunnel: w135 -> [w468 _]
      frame False {
      }
      frame True {
        n89 = local read "NOW date"() -> (→"date kickeron":string)
        n90 = local read "NOW time"() -> (→"time kickeron":string)
      }
    }
    n91 = Wait Until Next ms Multiple(millisecond multiple=u32 1000) -> ()  [unwired: 1 out]
    n92 = local read "date kickeron"() -> (w144:string)
    n93 = local read "time kickeron"() -> (w143:string)
    n94 = Get Date/Time In Seconds() -> (seconds since 1Jan1904=w260:timestamp)
    n95 = call-poly <userlib>:"CaLabGet.vi"("PV Names"=w23) -> ("1rst Value (string)"=w12:string[])  [unwired: 8 in, 6 out]
    n96 = Format Date/Time String(time format string (%c)="%Y/%m/%d", seconds (now)=w260) -> (date/time string=→"NOW date":string)  [unwired: 1 in]
    n97 = Format Date/Time String(time format string (%c)="%Y/%m/%d", seconds (now)=w260) -> (date/time string=w166:string)  [unwired: 1 in]
    n98 = Format Date/Time String(time format string (%c)="%H:%M:%S", seconds (now)=w260) -> (date/time string=w165:string)  [unwired: 1 in]
    "NOW time" <- w165
    n99 = Index Array(array=w12, index #1=0 ("index"), index #2=1 ("index"), index #3=2 ("index"), index #4=3 ("index"), index #5=4 ("index"), index #6=5 ("index"), index #7=6 ("index"), index #8=7 ("index"), index #9=8 ("index"), index #10=9 ("index")) -> (element #1=w11:string, element #2=w10:string, element #3=w9:string, element #4=w8:string, element #5=w7:string, element #6=w6:string, element #7=w5:string, element #8=w4:string, element #9=w3:string, element #10=w2:string)
    n100 = Bundle By Name(cluster=T1 {"SR Fill Pattern"=array[864 elements], "Beam Current(mA"=301.620555, "Beam Lifetime(min)"=770.7265563058899, "Beamsize X(um)"=56.5710156889631, "Beamsize Y(um)"=33.98058018201897, "Tune X(from BPM)"=0.0, "Tune Y(from BPM)"=0.0, "Mode"="Top-Up", "NuX(from BBF) "=0.16718639681347974, "NuY(from BBF)"=0.25229006370018453, "IU22-23gap(R)"=11.0, "IU22-05gap(R)"=7.791, "IU22-05M"=TRUE, "IU22A-09gap(R)"=8.92, "IU22A-09M"=TRUE, "IU22B-09gap(R)"=40.001, "IU22B-09M"=FALSE, "IUT22-21gap(R)"=7.0, "IUT22-21M"=TRUE, "IU22-23M"=TRUE, "IU22A-25gap(R)"=7.0, "IU22A-25M"=TRUE, "IU22B-25gap(R)"=40.0, "IU22B-25M"=FALSE, "EPU48A-41gap(R)"=64.9992, "EPU48A-41gM"=FALSE, "EPU48B-41gap(R)"=65.00435, "EPU48B-41gM"=FALSE, "EPU46-45gap(R)"=39.99995, "EPU46-45gM"=TRUE, "EPU48A-41phase(R)"=0.0001, "EPU48B-41phase(R)"=0.0006500000000000001, "EPU46-45phase(R)"=-0.00315, "Grid volt.(V)(S)"=33.0, "Gun mode"="MBM", "Mod.3 HV(kV)(S)"=34.919999999999945, "SR"="SR_DMB_2016_1102_1124LOCO.data", "BR"="Booster_JT_2016_1129_1130.data", "Linac"="Linac2016_1005_0935.data", "LTB"="LTB_JT_2016_1005_1200.data", "BTS"="BTS_2016_1201_0900.data", "RF2 remote"=TRUE, "RF2 OP mode"=TRUE, "RF2 phase.(S)"=-59.19999999999999, "RF Freq.(s)"=499654671.97859037, "RF2 gap volt.(S)"=1400.0, "RF3 remote"=TRUE, "RF3 OP mode"=TRUE, "RF3 phase.(S)"=155.0, "RF3 gap volt.(S)"=1400.0, "BBF V"=TRUE, "BBF H"=TRUE, "BR ext. kicker1(kV)"=18.966, "BR ext. kicker2(kV)"=17.666, "BR ext. sep.1(V)"=318.8444, "BR ext. sep.2(V)"=444.5, "BR inj. sep.(V)"=105.19999999999999, "BR inj. kicker(kV)"=16.400000000000002, "SR kicker4(kV)"=8.354, "SR kicker3(kV)"=8.274, "SR kicker2(kV)"=8.314, "SR kicker1(kV)"=8.5, "SR inj. sep.2(V)"=417.0, "SR inj. sep.1(V)"=419.34160000000026, "Bucket Start"=100.0, "Bucket Last"=630.0, "Bucket Step"=10.0, "Orbit ILK(P)"=FALSE, "IU22-05 Hutch Enable"=TRUE, "IU22A-09M Hutch Enable"=TRUE, "IUT22-21M Hutch Enable"=TRUE, "IU22-23M Hutch Enable"=FALSE, "IU22A-25M Hutch Enable"=TRUE, "EPU48A-41M Hutch Enable"=FALSE, "EPU46-45M Hutch Enable"=TRUE, "EPU46-45 FE Enable"=TRUE, "EPU48A-41 FE Enable"=FALSE, "IU22A-25 FE Enable"=TRUE, "IU22-23 FE Enable"=FALSE, "IUT22-21 FE Enable"=TRUE, "IU22A-09 FE Enable"=TRUE, "IU22-05 FE Enable"=TRUE, "EPU48A-41pM"=TRUE, "EPU48B-41pM"=FALSE, "EPU46-45pM"=FALSE, "Gun volt.(V)(S)"=23.5, "Width count"=30.0, "2ns step"=2.0, "10ps delay"=100.0, "phase shifter"=130.00060000000002, "Taper"=1.0899999999999999, "05XBPMX 1"=120.119, "09XBPMX 1"=501.669, "21XBPMX 1"=620.577, "23XBPMX 1"=-41.877, "25XBPMX 1"=406.91700000000003, "41XBPMX 1"=359.778, "45XBPMX 1"=-128.568, "05XBPMY 1"=-63.622, "09XBPMY 1"=51.52, "21XBPMY 1"=-49.721000000000004, "23XBPMY 1"=-43.219, "25XBPMY 1"=404.32300000000004, "41XBPMY 1"=-96.095, "45XBPMY 1"=-15.115, "FOFB H"="On", "FOFB V"="On", "time string"="16:34:30", "date"="2016/12/03", "date (last kicker ON)"="wait to fire", "time string (last kicker ON)"="kickers", "BPMX Graph"={[1, 2, 3, 4, 5, 6, 7, 8, 9, 10, 11, 12, 13, 14, 15, 16, 17, 18, 19, 20, 21, 22, 23, 24, 25, 26, 27, 28, 29, 30, 31, 32, 33, 34, 35, 36, 37, 38, 39, 40, 41, 42, 43, 44, 45, 46, 47, 48, 49, 50, 51, 52, 53, 54, 55, 56, 57, 58, 59, 60, 61, 62, 63, 64, 65, 66, 67, 68, 69, 70, 71, 72, 73, 74, 75, 76, 77, 78, 79, 80, 81, 82, 83, 84, 85, 86, 87, 88, 89, 90, 91, 92, 93, 94, 95, 96, 97, 98, 99, 100, 101, 102, 103, 104, 105, 106, 107, 108, 109, 110, 111, 112, 113, 114, 115, 116, 117, 118, 119, 120, 121, 122, 123, 124, 125, 126, 127, 128, 129, 130, 131, 132, 133, 134, 135, 136, 137, 138, 139, 140, 141, 142, 143, 144, 145, 146, 147, 148, 149, 150, 151, 152, 153, 154, 155, 156, 157, 158, 159, 160, 161, 162, 163, 164, 165, 166, 167, 168, 169, 170, 171, 172, 173, 174], "1rst Value (number)"=[-43.296, 19.934, -65.391, -6.814, 81.632, -64.642, 59.879, -27.142, 39.754, -58.914, 80.056, -31.919, -162.598, 0.751, 4.345, -254.365, -59.641, -21.912, 78.986, -87.374, 93.671, -23.166, 29.418, -120.78, -65.035, 169.371, 222.351, 229.913, -29.461000000000002, 64.357, 606.939, 477.06, -112.56700000000001, -49.853, 158.304, -60.217, -3.133, 38.6, -29.538, -130.835, -29.684, 141.751, -66.812, 43.146, 29.66, -18.359, -90.014, -19.177, 106.96600000000001, -89.0, 47.678000000000004, 96.199, -13.614, -177.47, 70.284, 64.789, -105.934, 66.406, 14.762, -23.425, -118.827, 6.7410000000000005, 102.941, -47.401, 47.422000000000004, -60.287, 37.002, -49.495000000000005, 40.904, -26.044, -238.314, -12.971, -318.762, -217.132, -130.297, 87.56400000000001, -21.939, -22.650000000000002, 64.413, -108.632, 77.42, -78.054, 10.784, -4.28, -527.735, -137.586, -297.907, -154.01, 142.577, 120.346, -68.403, 26.178, 27.319, -112.494, 164.46200000000002, 49.339, -58.179, -49.501, 9.484, 35.14, -114.35900000000001, 127.308, 34.477000000000004, -26.181, -113.21900000000001, 35.018, 37.901, -126.884, 139.51500000000001, 34.091, -38.265, -96.122, -10.536, 96.896, -86.46600000000001, 45.765, 70.086, -66.547, -117.522, 9.733, 88.72200000000001, -51.309000000000005, 46.455, 25.218, -31.145, -38.923, 23.922, 0.34700000000000003, -162.758, 172.109, 198.127, -181.357, -44.662, 14.011000000000001, -14.808, -71.82600000000001, 68.441, -39.97, 19.973, -54.454, -34.911, 61.058, 54.268, 143.52700000000002, -219.591, -297.907, 179.81300000000002, 72.425, -134.917, 49.111000000000004, 29.809, -59.177, 50.92, 27.761, -16.929000000000002, -77.932, -6.2170000000000005, 113.739, -134.417, 139.468, -4.478, -7.994, -120.53, -1.8940000000000001, 129.001, -113.745, 91.746, 39.779, -26.328, -129.276, 21.731, 89.459, -34.302, 10.308]}, "BPMY Graph"={[1, 2, 3, 4, 5, 6, 7, 8, 9, 10, 11, 12, 13, 14, 15, 16, 17, 18, 19, 20, 21, 22, 23, 24, 25, 26, 27, 28, 29, 30, 31, 32, 33, 34, 35, 36, 37, 38, 39, 40, 41, 42, 43, 44, 45, 46, 47, 48, 49, 50, 51, 52, 53, 54, 55, 56, 57, 58, 59, 60, 61, 62, 63, 64, 65, 66, 67, 68, 69, 70, 71, 72, 73, 74, 75, 76, 77, 78, 79, 80, 81, 82, 83, 84, 85, 86, 87, 88, 89, 90, 91, 92, 93, 94, 95, 96, 97, 98, 99, 100, 101, 102, 103, 104, 105, 106, 107, 108, 109, 110, 111, 112, 113, 114, 115, 116, 117, 118, 119, 120, 121, 122, 123, 124, 125, 126, 127, 128, 129, 130, 131, 132, 133, 134, 135, 136, 137, 138, 139, 140, 141, 142, 143, 144, 145, 146, 147, 148, 149, 150, 151, 152, 153, 154, 155, 156, 157, 158, 159, 160, 161, 162, 163, 164, 165, 166, 167, 168, 169, 170, 171, 172, 173, 174], "1rst Value (number)"=[-162.203, -14.73, -4.856, 96.402, -32.102000000000004, -4.38, 27.845, -16.177, 4.523, 0.355, -59.075, 8.066, -8.208, 1.3820000000000001, -3.302, 54.915, -4.521, -26.793, 34.564, -24.867, 12.514000000000001, 47.257, -94.551, 6.994, 53.555, -32.288000000000004, 23.119, 31.675, -210.978, -77.309, 164.597, 56.306000000000004, 49.414, -23.167, -22.805, -4.821, -5.111, -24.758, 36.562, 20.89, -33.417, 25.87, 33.105000000000004, 13.876, 8.116, -27.615000000000002, 5.676, 7.4, -34.08, 4.7860000000000005, -31.904, 20.297, 8.358, -7.194, 42.963, 18.578, -84.399, 52.552, -81.0, 93.979, -68.614, 15.918000000000001, -39.702, 52.068, -52.719, 50.638, -35.623, 7.589, 44.783, -42.32, 76.897, 9.802, -167.399, -69.894, 6.93, 7.448, 11.853, -51.636, 35.626, 16.401, 15.221, 13.867, 48.198, -29.538, 32.547000000000004, 2.207, -10.84, -113.852, 120.884, -37.52, 42.201, 3.6, 13.983, -3.926, 19.779, -10.033, -10.826, -13.336, 31.166, -39.277, 0.343, 6.99, -29.462, 58.393, -2.8000000000000003, -26.037, 22.0, -13.565, -2.559, 3.5740000000000003, -24.974, -1.725, 27.884, -44.505, 51.879, -29.419, 12.565, 41.444, 15.836, 10.574, -2.486, 17.956, -26.659, -7.453, -10.4, 19.556, -6.492, -30.583000000000002, -45.81, -19.923000000000002, -6.239, -9.737, 12.615, -28.353, -29.506, 62.644, -32.28, -1.966, 3.197, -7.515000000000001, 52.962, -47.023, 39.379, 36.821, 88.622, 12.058, 7.498, 111.892, -47.882, 17.074, -31.824, 12.244, 30.484, -19.358, -1.157, 10.999, 1.948, -22.885, -7.635, 11.559000000000001, -9.788, -11.97, -3.1, 26.501, 6.728, -26.645, 6.832, 76.879, -121.083, 38.427, 9.151, -12.502, 33.426, -2.866]}, "Radio Buttons 2"=enum."absolute", "09XBPMX 2"=" PAB ", "09XBPMY 2"=" closed", "05XBPMY 2"="-172.06", "05XBPMX 2"="-641.02", "21XBPMY 2"="-530.88", "21XBPMX 2"="-953.53", "23XBPMY 2"=" closed", "23XBPMX 2"="FE ", "25XBPMY 2"="1498.85", "25XBPMX 2"="138.49", "41XBPMY 2"=" closed", "41XBPMX 2"="FE ", "45XBPMX 2"=" PAB ", "45XBPMY 2"=" closed", "05 mode"="Follow", "09A mode"="Follow", "09B mode"="Follow", "21 mode"="Follow", "23 mode"="Follow", "25A mode"="Follow", "25B mode"="Follow", "41A mode"="Follow", "41B mode"="Follow", "46 mode"="Follow"} ("Cluster"), "Tune X(from BPM)"=w138, "Tune Y(from BPM)"=w137, "date (last kicker ON)"=w144, "time string (last kicker ON)"=w143, "date"=w166, "time string"=w165, "Mode"=w251, "Beam Current(mA"=w250, "Beam Lifetime(min)"=w249, "Beamsize X(um)"=w248, "Beamsize Y(um)"=w247, "NuX(from BBF)"=w246, "NuY(from BBF)"=w245, "Bucket Start"=w244, "Bucket Last"=w243, "Bucket Step"=w242, "BR inj. sep.(V)"=w241, "BR inj. kicker(kV)"=w240, "BR ext. kicker1(kV)"=w239, "BR ext. kicker2(kV)"=w238, "BR ext. sep.1(V)"=w237, "BR ext. sep.2(V)"=w236, "SR inj. sep.1(V)"=w235, "SR inj. sep.2(V)"=w234, "SR kicker1(kV)"=w233, "SR kicker2(kV)"=w232, "SR kicker3(kV)"=w231, "SR kicker4(kV)"=w230, "Gun mode"=w229, "Grid volt.(V)(S)"=w228, "Gun volt.(V)(S)"=w227, "Mod.3 HV(kV)(S)"=w226, "Width count"=w225, "2ns step"=w224, "10ps delay"=w223, "RF2 remote"=w222, "RF2 OP mode"=w221, "RF2 phase.(S)"=w142, "RF Freq.(s)"=w220, "RF2 gap volt.(S)"=w141, "RF3 remote"=w219, "RF3 OP mode"=w218, "RF3 phase.(S)"=w217, "RF3 gap volt.(S)"=w216, "BR"=w215, "BTS"=w214, "Linac"=w212, "LTB"=w211, "SR"=w213, "SR Fill Pattern"=w210, "IU22-05 Hutch Enable"=w87, "IU22A-09M Hutch Enable"=w83, "IUT22-21M Hutch Enable"=w67, "IU22-23M Hutch Enable"=w50, "IU22A-25M Hutch Enable"=w49, "EPU48A-41M Hutch Enable"=w31, "EPU46-45M Hutch Enable"=w30, "EPU46-45 FE Enable"=w32, "EPU48A-41 FE Enable"=w33, "IU22A-25 FE Enable"=w51, "IU22-23 FE Enable"=w52, "IUT22-21 FE Enable"=w70, "IU22A-09 FE Enable"=w82, "IU22-05 FE Enable"=w88, "IU22-05gap(R)"=w209, "IU22A-09gap(R)"=w208, "IU22B-09gap(R)"=w207, "IUT22-21gap(R)"=w206, "IU22-23gap(R)"=w205, "IU22A-25gap(R)"=w204, "IU22B-25gap(R)"=w203, "EPU48A-41gap(R)"=w202, "EPU48A-41phase(R)"=w201, "EPU48B-41gap(R)"=w200, "EPU48B-41phase(R)"=w199, "EPU46-45gap(R)"=w198, "EPU46-45phase(R)"=w197, "Taper"=w139, "phase shifter"=w196, "05XBPMX 1"=w195, "09XBPMX 1"=w194, "21XBPMX 1"=w193, "23XBPMX 1"=w192, "25XBPMX 1"=w191, "41XBPMX 1"=w190, "45XBPMX 1"=w189, "05XBPMY 1"=w188, "09XBPMY 1"=w187, "21XBPMY 1"=w186, "23XBPMY 1"=w185, "25XBPMY 1"=w184, "41XBPMY 1"=w183, "45XBPMY 1"=w182, "IU22-05M"=w181, "IU22A-09M"=w180, "IU22B-09M"=w179, "IUT22-21M"=w178, "IU22-23M"=w177, "IU22A-25M"=w176, "IU22B-25M"=w175, "EPU48A-41gM"=w174, "EPU48B-41gM"=w173, "EPU46-45gM"=w172, "EPU48A-41pM"=w171, "EPU48B-41pM"=w170, "EPU46-45pM"=w169, "BPMX Graph"=w168, "BPMY Graph"=w167, "Radio Buttons 2"=enum32{"absolute", "different with"}."absolute", "FOFB H"=w150, "FOFB V"=w149, "BBF H"=w148, "BBF V"=w147, "Orbit ILK(P)"=w146, "05XBPMX 2"=w77, "05XBPMY 2"=w76, "09XBPMX 2"=w75, "09XBPMY 2"=w74, "21XBPMX 2"=w59, "21XBPMY 2"=w58, "23XBPMX 2"=w57, "23XBPMY 2"=w56, "25XBPMX 2"=w39, "25XBPMY 2"=w38, "41XBPMX 2"=w37, "41XBPMY 2"=w36, "45XBPMX 2"=w35, "45XBPMY 2"=w34, "05 mode"=w11, "09A mode"=w10, "09B mode"=w9, "21 mode"=w8, "23 mode"=w7, "25A mode"=w6, "25B mode"=w5, "41A mode"=w4, "41B mode"=w3, "46 mode"=w2) -> (→"Cluster":T1)
  }
  n101 = while {
    i -> [w489]
    stop <- w487 stop-if-true
    # "D:\\LOG運轉紀錄\\2016"
    n102 = event shown="[0] Timeout" {
      selector: _ -> [_ _ _ _]
      dyn-events: _ -> [_ _ _ _]
      timeout: 233 -> [_ _ _ _]
      tunnel: [_ TRUE ("stop") _ _] -> w491
      event Timeout {
        n103 = event-data() -> ()  [unwired: 1 in, 3 out]
      }
      event "stop": Value Change {
        n104 = event-data() -> ()  [unwired: 1 in, 4 out]
      }
      event "Open Button": Value Change {
        n105 = event-data() -> ()  [unwired: 1 in, 6 out]
        n106 = Get Date/Time In Seconds() -> (seconds since 1Jan1904=w515:timestamp)
        n107 = Format Date/Time String(time format string (%c)="%Y", seconds (now)=w515, UTC format=FALSE) -> (date/time string=w507:string)
        n108 = Format Date/Time String(time format string (%c)="%d", seconds (now)=w515, UTC format=FALSE) -> (date/time string=w498:string)
        n109 = call "to_be_2_string.vi"("string 2"=w498) -> ("substring 2"=w497:string)  [unwired: 10 in]
        n110 = Format Date/Time String(time format string (%c)="%m", seconds (now)=w515, UTC format=FALSE) -> (date/time string=w503:string)
        n111 = Concatenate Strings("D" ("磁碟位置"), ":\\LOG運轉紀錄\\", w507, "\\", w503, "\\", w497) -> (w495:string)
        n112 = String To Path(string=w495) -> (path=w511:path)
        n113 = call <vilib>:"Check if File or Folder Exists.vi"("path"=w511) -> ("error out"=w513:errorcluster, "file or folder exists?"=w499:bool, "dup path"=w512:path)  [unwired: 8 in]
        n114 = case shown="False" w499 {
          tunnel: w512 -> [w522 w524]
          tunnel: w513 -> [w521 w523]
          tunnel: [w520 w524] -> _
          tunnel: [w519 w523] -> w496
          frame False {
            n115 = Create Folder(path (use dialog)=w522, error in=w521) -> (created path=w520:path, error out=w519:errorcluster)  [unwired: 1 in, 1 out]
          }
          frame True {
          }
        }
        n116 = Concatenate Strings("explorer ", w495) -> (w517:string)
        n117 = call <vilib>:"System Exec.vi"("wait until completion? (T)"=FALSE, "error in (no error)"=w496, "command line"=w517) -> ()  [unwired: 5 in, 4 out]
      }
      event "Save Button": Value Change {
        n118 = event-data() -> ()  [unwired: 1 in, 6 out]
        n119 = Get Date/Time In Seconds() -> (seconds since 1Jan1904=w554:timestamp)
        n120 = Format Date/Time String(time format string (%c)="%Y", seconds (now)=w554, UTC format=FALSE) -> (date/time string=w535:string)
        n121 = Format Date/Time String(time format string (%c)="%d", seconds (now)=w554, UTC format=FALSE) -> (date/time string=w526:string)
        n122 = call "to_be_2_string.vi"("string 2"=w526) -> ("substring 2"=w525:string)  [unwired: 10 in]
        n123 = Format Date/Time String(time format string (%c)="%m", seconds (now)=w554, UTC format=FALSE) -> (date/time string=w531:string)
        n124 = Format Date/Time String(time format string (%c)="%Y%m%d%H%M%S", seconds (now)=w554) -> (date/time string=w547:string)  [unwired: 1 in]
        n125 = Concatenate Strings("D" ("磁碟位置"), ":\\LOG運轉紀錄\\", w535, "\\", w531, "\\", w525) -> (w542:string)
        n126 = String To Path(string=w542) -> (path=w539:path)
        n127 = call <vilib>:"Check if File or Folder Exists.vi"("path"=w539) -> ("error out"=w541:errorcluster, "file or folder exists?"=w527:bool, "dup path"=w540:path)  [unwired: 8 in]
        n128 = invoke on="Cluster" class="Clust (strict)" method="Get Image"() -> ("image data"=w556:T2)  [unwired: 6 in, 5 out]
        n129 = case shown="False" w527 {
          tunnel: w540 -> [w560 w562]
          tunnel: w541 -> [w559 w561]
          tunnel: [w558 w562] -> w555
          tunnel: [w557 w561] -> _
          frame False {
            n130 = Create Folder(path (use dialog)=w560, error in=w559) -> (created path=w558:path, error out=w557:errorcluster)  [unwired: 1 in, 1 out]
          }
          frame True {
          }
        }
        n131 = Path To String(path=w555) -> (string=w543:string)
        n132 = Concatenate Strings(w543, "\\" ("string"), w547) -> (w553:string)
        n133 = Concatenate Strings(w553, ".jpg" ("file format")) -> (w552:string)
        n134 = String To Path(string=w552) -> (path=w548:path)
        n135 = call <vilib>:"Write JPEG File.vi"("quality (80)"=100, "image data"=w556, "path to JPEG file"=w548) -> ("error out"=→"error out 3":errorcluster)  [unwired: 7 in, 1 out]
      }
    }
    n136 = local read "stop"() -> (w492:bool)
    n137 = Or(x=w491, y=w492) -> (x .or. y?=w487:bool)
    n138 = case shown="True" TRUE {
      tunnel: w487 -> [_ w493]
      frame False {
      }
      frame True {
        n139 = Quit LabVIEW(quit? (T)=w493) -> ()
      }
    }
    "loop2" <- w489
  }
  n140 = local write "stop"(FALSE ("stop")) -> ()
